vi "Consumer.vi"(8 "error in (no error)":errorcluster, 9 "Data":variant, 10 "Case ID":string, 11 "Monkey in":refnum<class "Monkey.lvclass">) -> (0 "error out":errorcluster, 3 "Monkey out":refnum<class "Monkey.lvclass">)   [LabVIEW 2020, in "TALOS.lvlib" / "Monkey.lvlib" / "Monkey.lvclass"]
uses:
  Monkey.lvclass
  C:/LabVIEW Code/TALOS/talos/Ancestor/Ancestor/Ancestor.lvclass
  C:/LabVIEW Code/TALOS/talos/Father of all uServices/Father of all uServices/Father of all uServices.lvclass
  Monkey Consumer Case Selector.ctl
  Interfaces/Analysis Framework/Analysis Framework.lvclass
  Ancestor/Ancestor/Ancestor.lvclass/Ancestor.ctl
  Father of all uServices/Father of all uServices/Father of all uServices.lvclass/Father of all uServices.ctl
  Monkey.lvclass/Monkey.ctl
  Run Utilities/TypeDefs/Messages/Schedule Message.ctl
  Run Utilities/TypeDefs/DAQ Control.ctl
  Run Utilities/Schedule/Schedule.lvclass
  Father of all uServices/Father of all uServices Messages/Consumer Msg/Consumer Msg.lvclass/Consumer Msg.ctl
  Run Utilities/TypeDefs/Script Checker Result.ctl
  Run Utilities/TypeDefs/Messages/Script Checker Message.ctl
  Guardian/Guardian Messages/Message to uService Msg/Message to uService Msg.lvclass/Message to uService Msg.ctl
  Run Utilities/TypeDefs/Messages/Submit Message.ctl
  Run Utilities/Run Instance/Run Instance.lvclass
  Run Utilities/TypeDefs/Monkey Status.ctl
  Run Utilities/TypeDefs/Messages/Banana Message.ctl
  Run Utilities/TypeDefs/Return Code.ctl
  Inner stop message.ctl
  Ancestor/Ancestor/Read ID.vi
  Guardian/Guardian Messages/Message to uService Msg/Send Message to uService.vi
  FGV/Error Memory/Get Error Description.vi
  Support VIs/Get PC name.vi
  Support VIs/Get Class Name.vi
  FGV/Error Memory/Error Memory Core.vi
  <vilib>/AdvancedString/Delimited String to 1D String Array.vi
  Support VIs/Circus Root Path.vi
  FGV/Error Memory/Error Crt Lvl checker.vi
  FGV/Error Memory/Error Memory Core.vi/40c8088d-b597-4017-91af-faa98e00292e.vi
  FGV/Error Memory/Error Memory Core.vi/d4a3ab98-063c-4e44-b43d-fbdcfe6c2be2.vi
  Father of all uServices/Father of all uServices/Father of all uServices.lvclass
  C:/LabVIEW Code/TALOS/builds/Actor Framework PPL/Actor Framework.lvlibp/1abvi3w/vi.lib/ActorFramework/Actor/Actor.lvclass
  Run Utilities/Optimiser Cell/Optimiser Cell.lvclass
  C:/LabVIEW Code/TALOS/talos/Run Utilities/Cell/Schedule Cell.lvclass
  Support VIs/Global Memory.vi
  <vilib>/Utility/LVClass/Get LV Class Name.vi
  Support VIs/Is in Packed Library.vi
  Support VIs/TALOS Root path.vi
  Support VIs/Read CSV worksheet.vi
  Support VIs/Global Constants.vi
  <vilib>/Utility/error.llb/General Error Handler.vi
  <vilib>/Utility/config.llb/Open Config Data.vi
  <vilib>/Utility/config.llb/Get Section Names.vi
  <vilib>/Utility/config.llb/Get Key Names.vi
  <vilib>/Utility/config.llb/Read Key.vi
  <vilib>/Utility/config.llb/Read Key (String).vi
  <vilib>/Utility/config.llb/Close Config Data.vi
  <vilib>/Utility/error.llb/Search and Replace Pattern.vi
  Support VIs/Error Log.vi
  builds/Actor Framework PPL/Actor Framework.lvlibp/1abvi3w/vi.lib/ActorFramework/Actor/Read Self Enqueuer.vi
  <userlib>/_OpenG.lib/lvdata/lvdata.llb/Get Strings from Enum__ogtk.vi
  builds/Actor Framework PPL/Actor Framework.lvlibp/1abvi3w/vi.lib/ActorFramework/Message Enqueuer/Enqueue.vi
  builds/Actor Framework PPL/Actor Framework.lvlibp/1abvi3w/vi.lib/ActorFramework/Actor/Read Caller Enqueuer.vi
  Father of all uServices/Father of all uServices/Children Methods/Get GUI Item Value - String.vi
  Father of all uServices/Father of all uServices/Multiline string updater.vi
  Ancestor/Ancestor/Ancestor.lvclass
  <vilib>/Comparison/Equal/Equal Functor/Equal Functor.lvclass
  Father of all uServices/Father of all uServices Messages/Consumer Msg/Consumer Msg.lvclass
  Run Utilities/Run Block/Run Block.lvclass
  Guardian/Guardian Messages/Message to uService Msg/Message to uService Msg.lvclass
  TALOS.lvlib
  Run Utilities/Run Utilities.lvlib
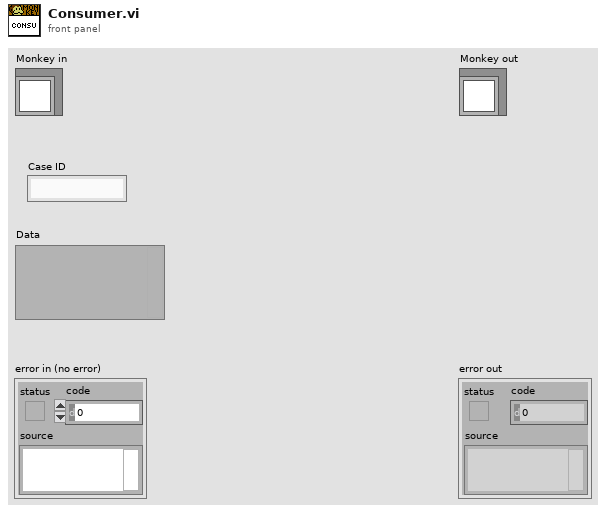
[diagram p1: front panel]
types:
  T1 = typedef "TALOS.lvlib/Monkey.lvlib/Monkey.lvclass/Monkey Consumer Case Selector.ctl" = enum16{"Init", "Update GUI", "New schedule", "Check Script", "Submit Script", "Banana arrived", "Optimiser - evaluate RUN", "Optimiser - update RUN", "Quality Check", "What to do next", "Update Crit Lvl", "Skip Run", "Stop Schedule", "Skip schedule"}
  T2 = cluster{"Font Name:":string, "Size":i16, "Strikeout?":bool, "Italic?":bool, "Underline?":bool, "Outline?":bool, "Shadow?":bool, "Bold?":bool}
  T3 = enum16{"User-specified Font", "Application Font", "System Font", "Dialog Font"}
  T4 = typedef "TALOS.lvlib/Run Utilities.lvlib/Schedule Message.ctl" = cluster{"uS Name":string, "Synchronised":bool, "DAQ Control":T5, "Schedule":refnum<class "Schedule.lvclass">}
  T5 = typedef "TALOS.lvlib/Run Utilities.lvlib/DAQ Control.ctl" = enum16{"On", "Off", "External"}
  T6 = typedef "TALOS.lvlib/Run Utilities.lvlib/Script Checker Message.ctl" = cluster{"Monkey ID":string, "Script Checker Result":T7}
  T7 = typedef "TALOS.lvlib/Run Utilities.lvlib/Script Checker Result.ctl" = enum16{"Passed", "Failed", "Empty"}
  T8 = typedef "TALOS.lvlib/Run Utilities.lvlib/Monkey Status.ctl" = enum16{"Init", "Paused", "Ongoing", "Stopped", "Finished (no errors)", "Finished (with errors)"}
  T9 = typedef "TALOS.lvlib/Run Utilities.lvlib/Submit Message.ctl" = cluster{"DAQ Control":T5, "Run Instance":refnum<class "Run Instance.lvclass">}
  T10 = typedef "TALOS.lvlib/Run Utilities.lvlib/Banana Message.ctl" = cluster{"FPGA Name":string, "Return Code":T11}
  T11 = typedef "TALOS.lvlib/Run Utilities.lvlib/Return Code.ctl" = enum16{"All Good", "Retry", "Skip", "Skip All", "ABORT"}
  T12 = cluster{"left":i16, "top":i16, "right":i16, "bottom":i16}
  T13 = typedef "TALOS.lvlib/Run Utilities.lvlib/Run Instance.lvclass/Run Instance - GUI.ctl" = cluster{"Script Name":string, "Parameters":string[][], "FPGA Name":string}
  T14 = typedef "TALOS.lvlib/Run Utilities.lvlib/Schedule.lvclass/Array of Runs - GUI.ctl" = T15[]
  T15 = typedef "TALOS.lvlib/Run Utilities.lvlib/Schedule Cell.lvclass/Cell - GUI.ctl" = cluster{"Background Color":u32, "Number of cycles":u32, "Single RUN":T13, "Quality check":bool, "Cell Type":string}
  T16 = typedef "TALOS.lvlib/Monkey.lvlib/Monkey.lvclass/Inner stop message.ctl" = cluster{"Old value":bool, "Gracefully?":bool}
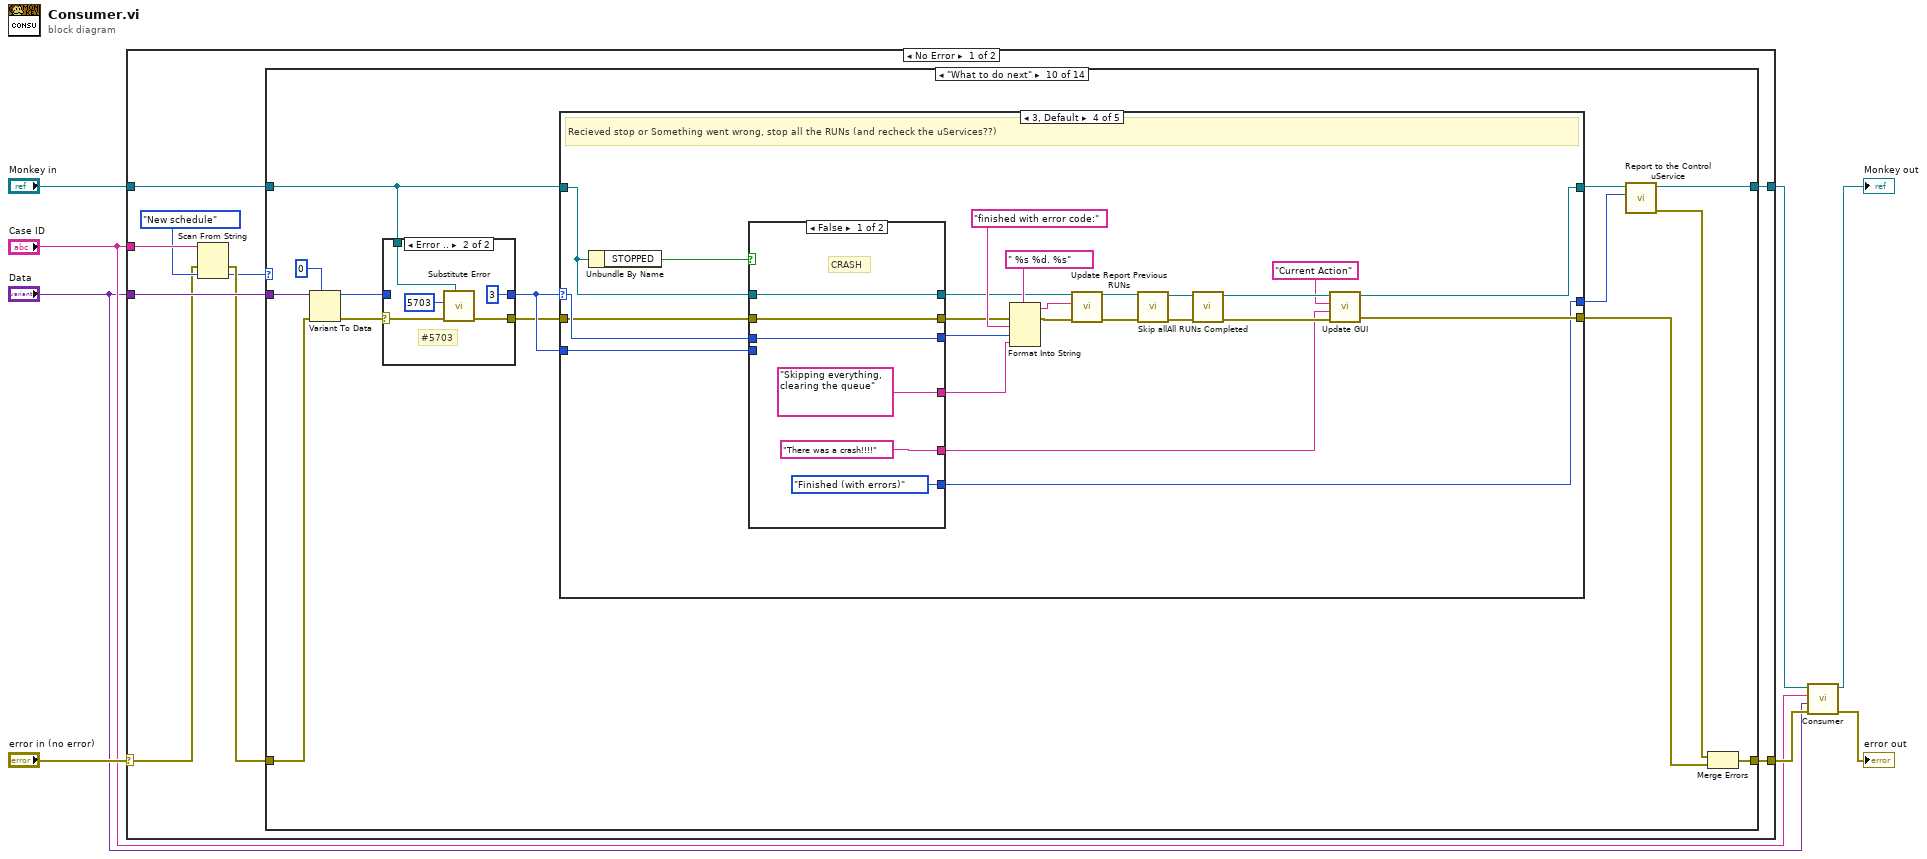
[diagram p0: block diagram]
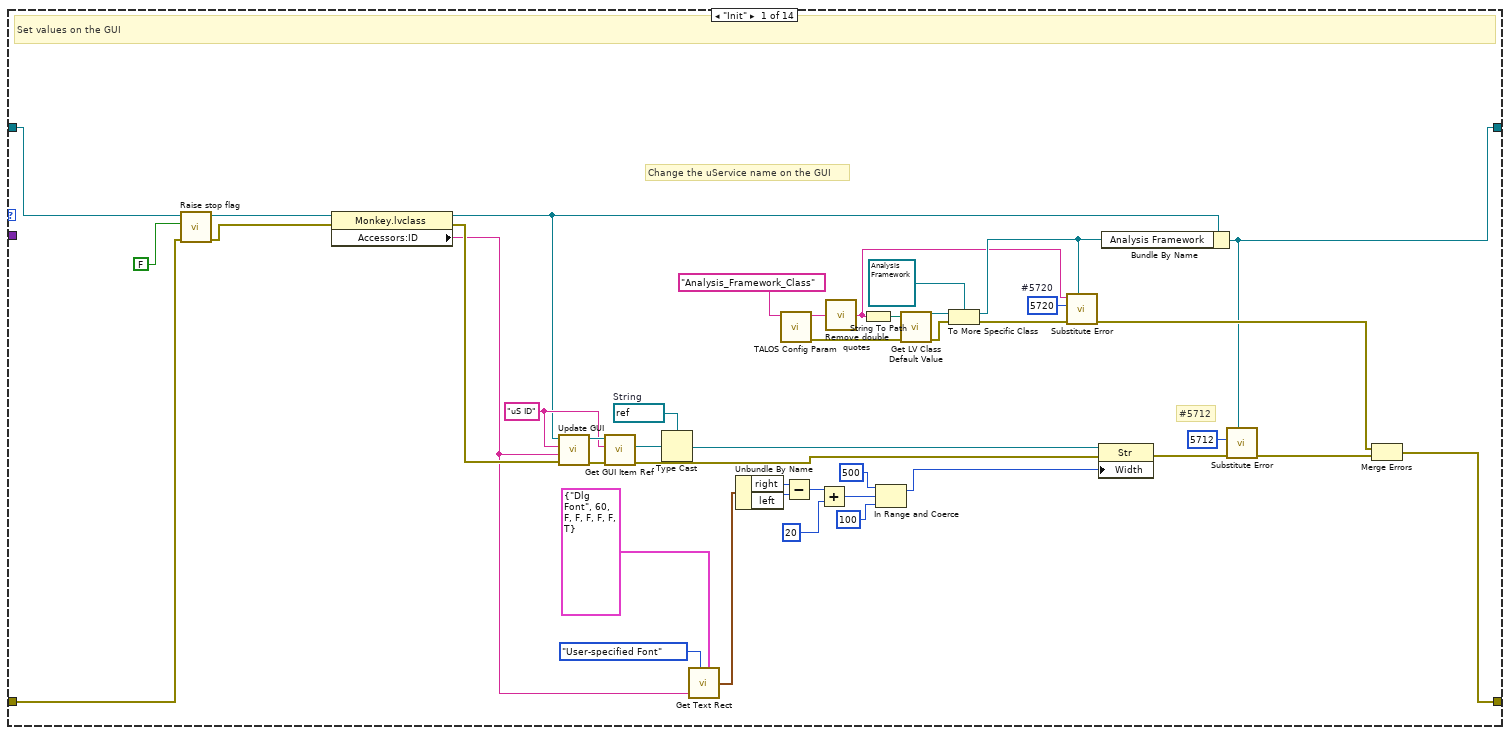
[diagram p2: hidden frame]
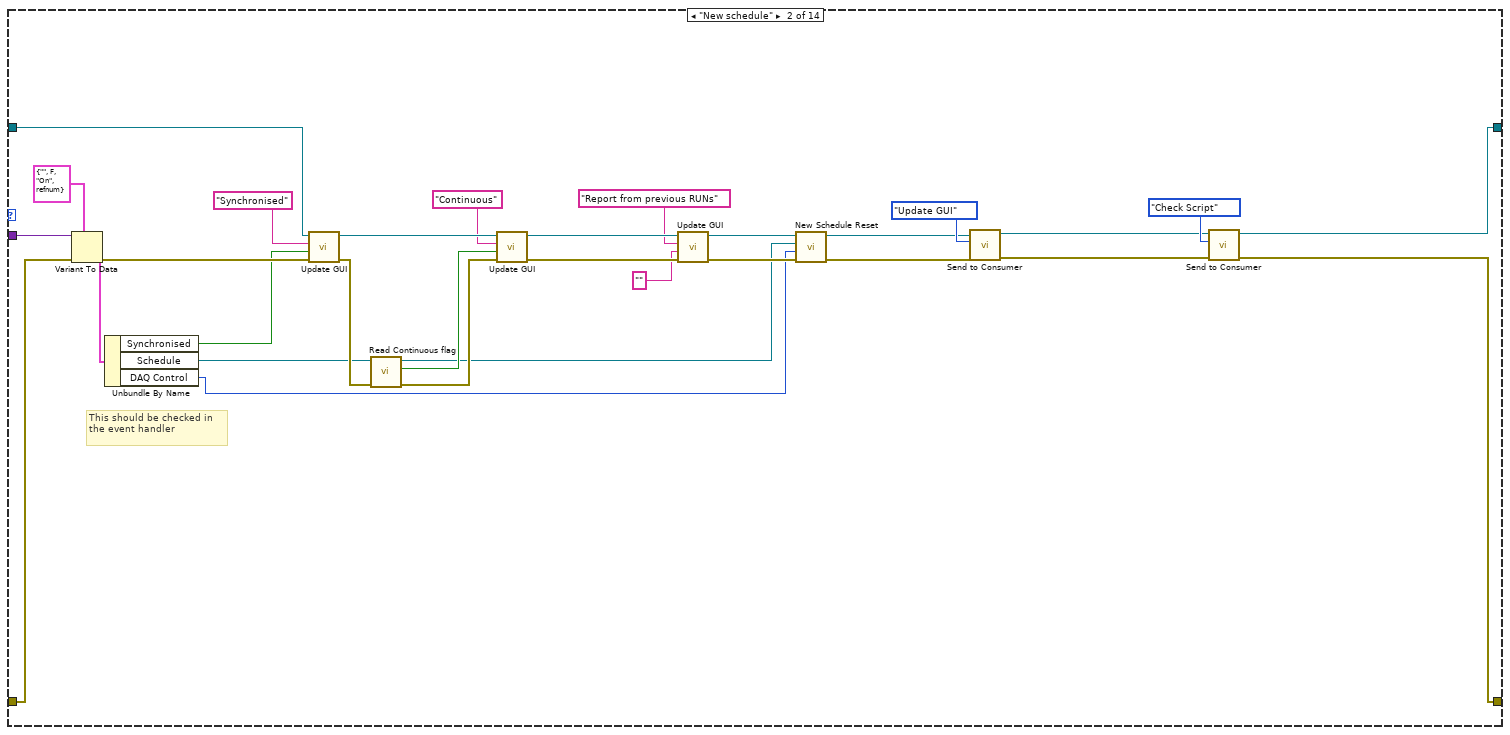
[diagram p3: hidden frame]
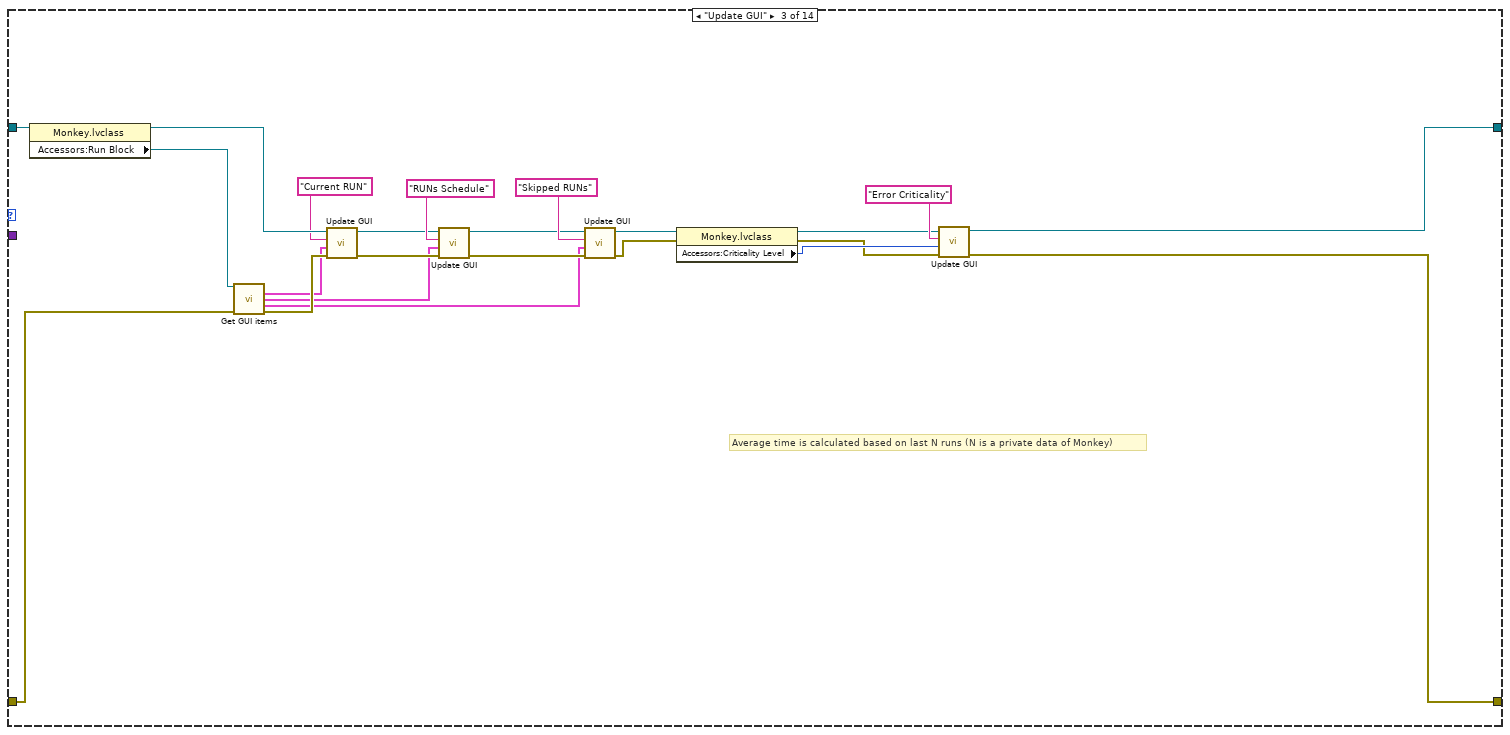
[diagram p4: hidden frame]
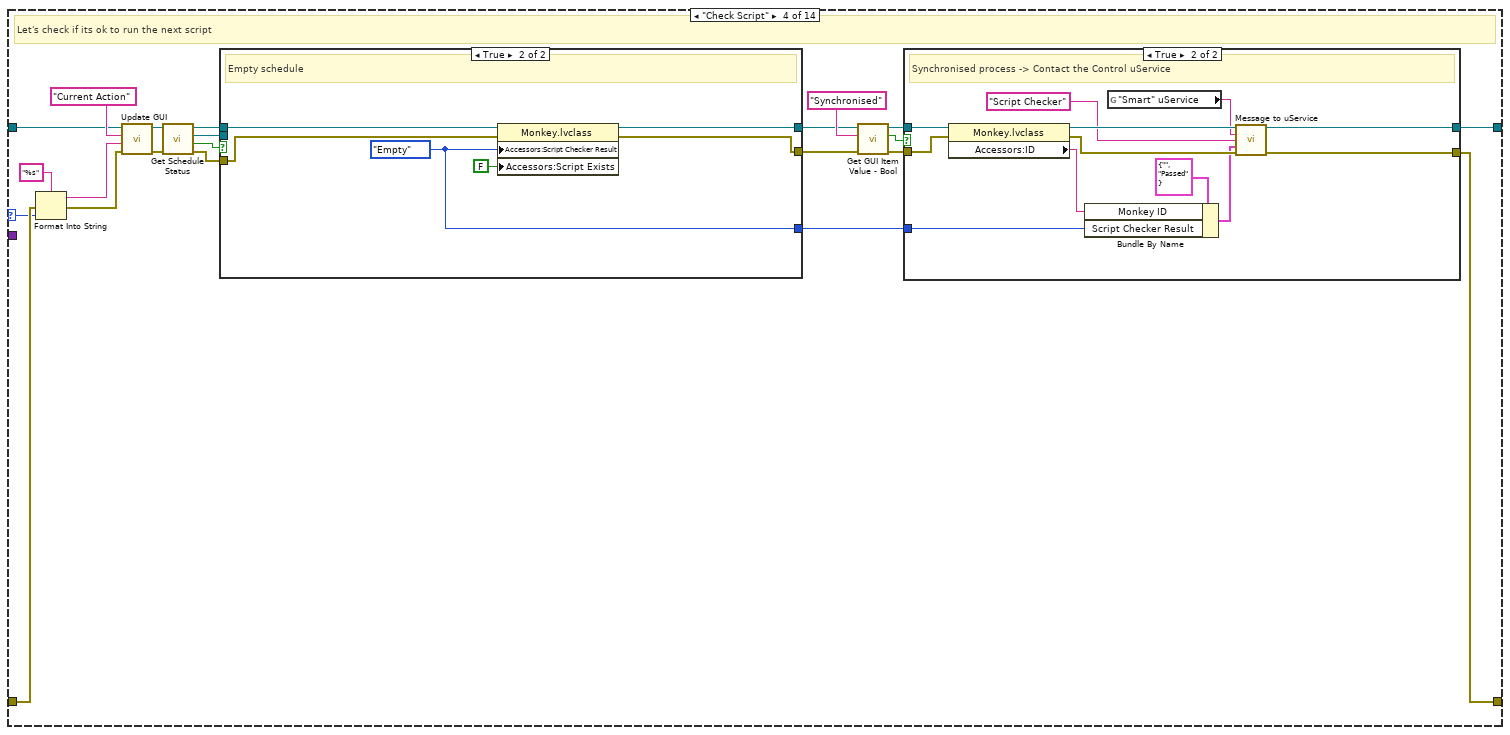
[diagram p5: hidden frame]
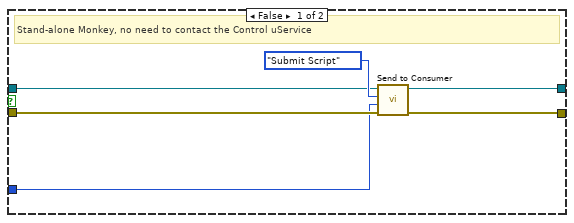
[diagram p6: hidden frame]
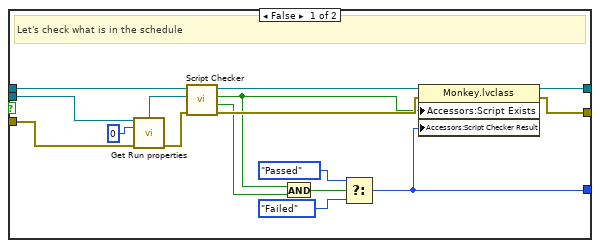
[diagram p7: hidden frame]
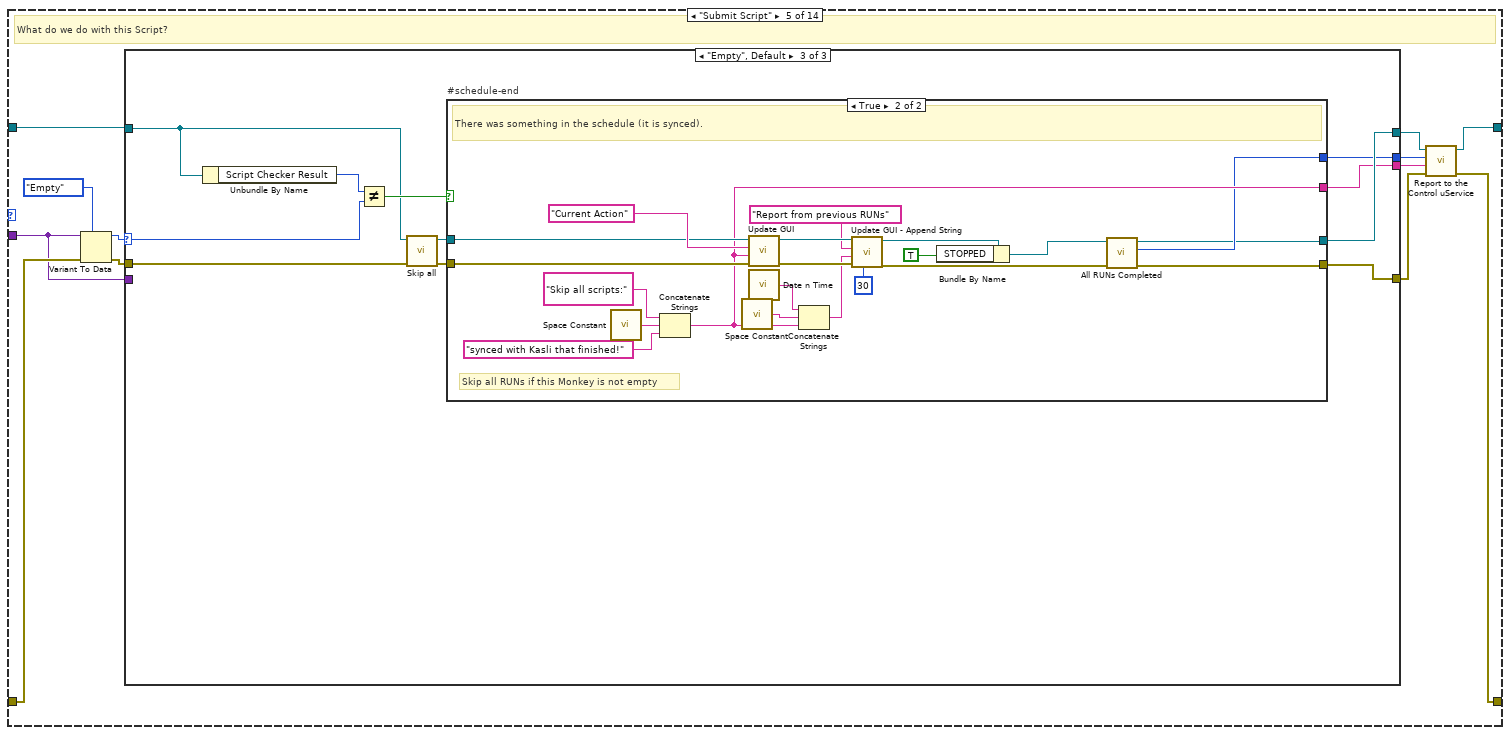
[diagram p8: hidden frame]
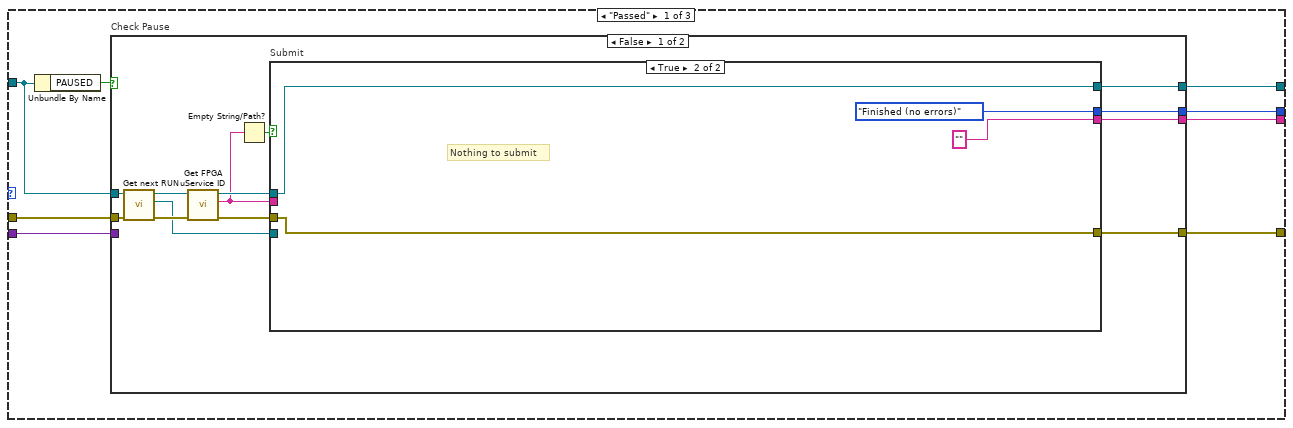
[diagram p9: hidden frame]
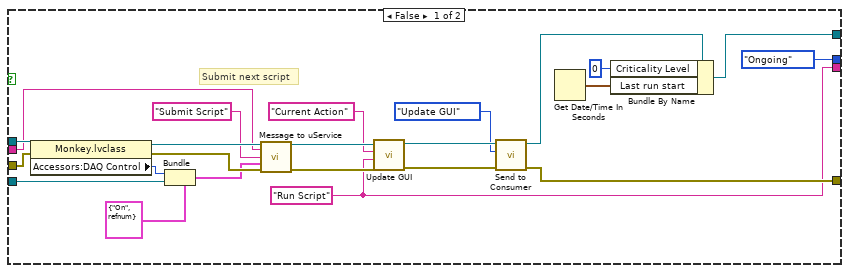
[diagram p10: hidden frame]
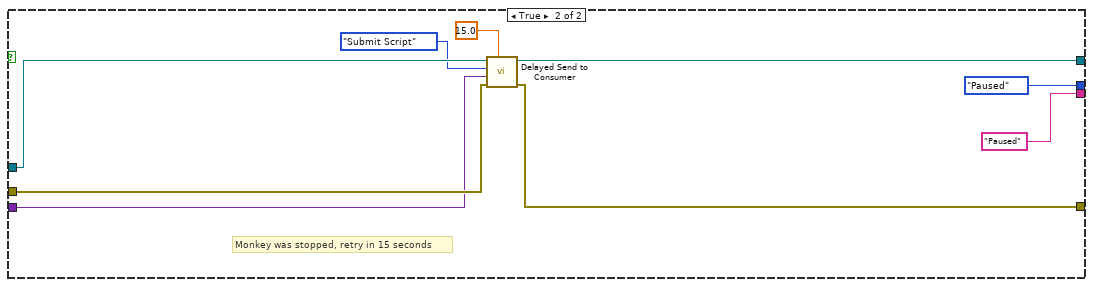
[diagram p11: hidden frame]
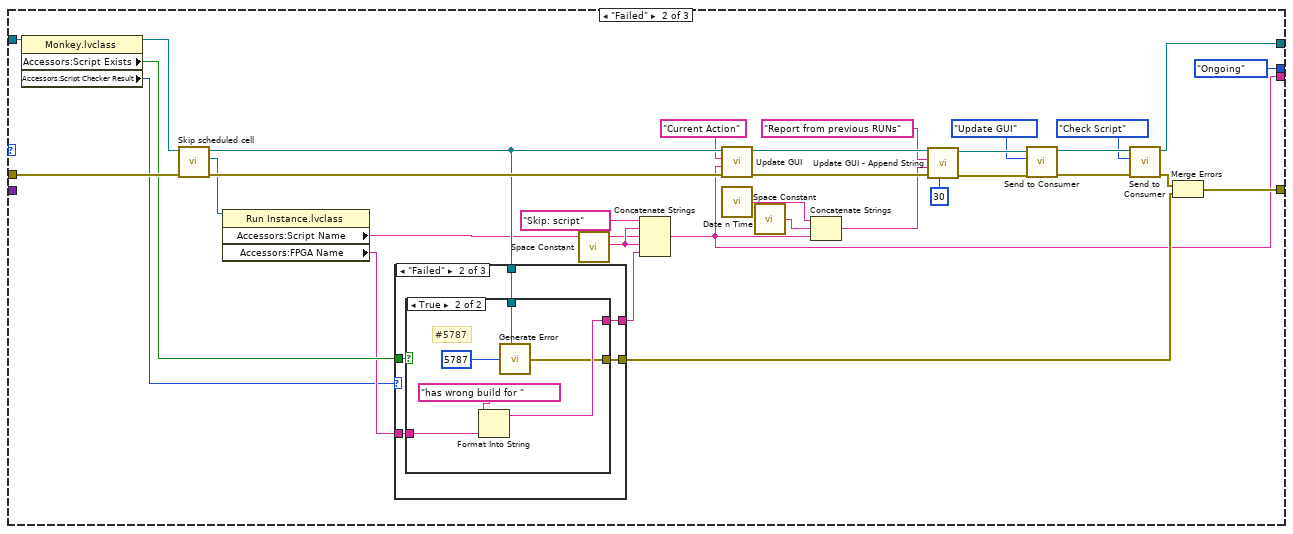
[diagram p12: hidden frame]
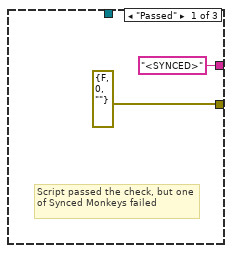
[diagram p13: hidden frame]
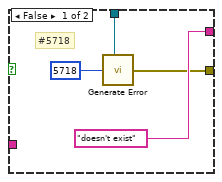
[diagram p14: hidden frame]
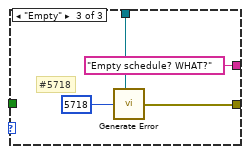
[diagram p15: hidden frame]
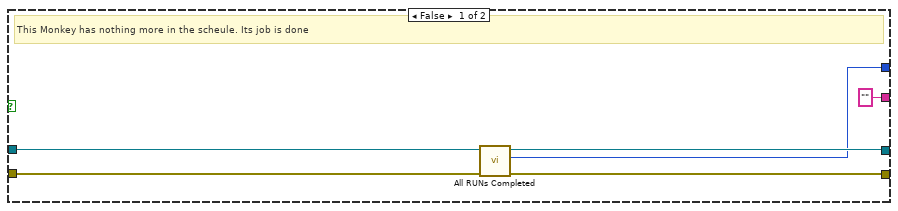
[diagram p16: hidden frame]
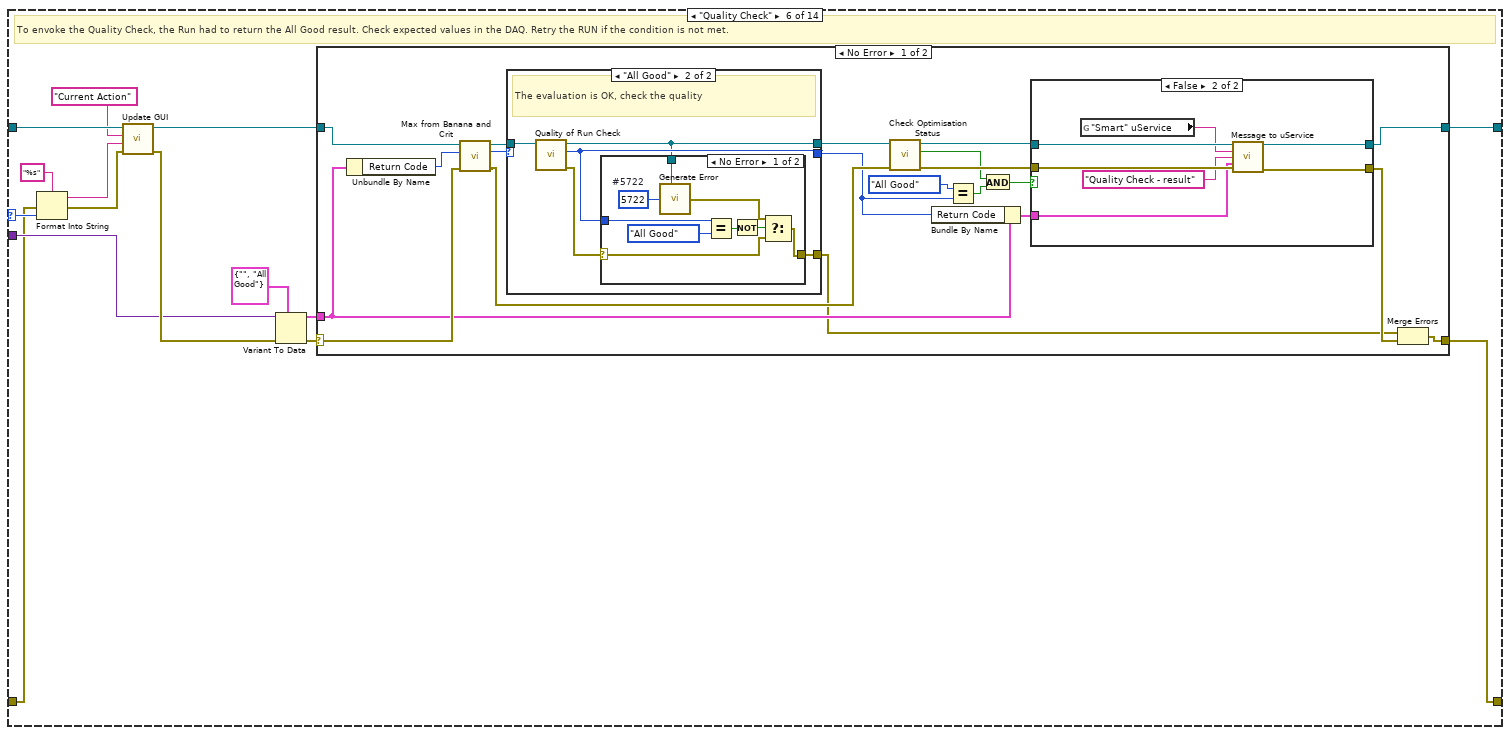
[diagram p17: hidden frame]
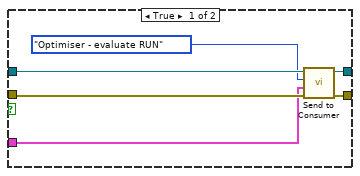
[diagram p18: hidden frame]
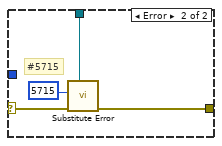
[diagram p20: hidden frame]
diagram:
  n1 = case shown="No Error" "error in (no error)" {
    selector: "error in (no error)" -> [w11 w975]
    tunnel: [w16 w976] -> w3
    tunnel: "Monkey in" -> [w17 w976]
    tunnel: [w14 w975] -> w6
    tunnel: "Case ID" -> [w13 _]
    tunnel: "Data" -> [w15 _]
    frame No Error {
      n2 = Scan From String(input string=w13, error in=w11, default 1=Monkey_Consumer_Case_Selector."New schedule" ("Consumer Case Selector")) -> (error out=w10:errorcluster, output 1=w9:T1)  [unwired: 2 in, 2 out]
      n3 = case shown="\"What to do next\"" w9 {
        selector: w9 -> [_ _ _ w114 _ w342 _ _ _ _ _ _ _ _]
        tunnel: w17 -> [w25 w78 w108 w116 w187 w350 w431 w523 w598 w627 w845 w880 w920 w974]
        tunnel: [w27 w62 w98 w125 w181 w348 w429 w520 w600 w629 w855 w883 w929 w964] -> w16
        tunnel: w15 -> [_ w87 _ _ w176 w349 w428 w519 w596 w631 w860 w884 w930 _]
        tunnel: [w30 w61 w97 w124 w179 w337 w430 w521 w599 w628 w854 w882 w928 w965] -> w14
        tunnel: w10 -> [w23 w84 w111 w118 w186 w339 w432 w522 w597 w630 w859 w890 w932 w973]
        frame "Init" {
          w32 = 5720  # #5720
          w55 = refnum<vi> refnum  # String
          w58 = "uS ID" ("GUI Item Name")
          # "Change the uService name on the GUI"
          # "#5712"
          # "Set values on the GUI"
          n4 = call-dynamic "Raise stop flag.vi"("error in (no error)"=w23, "on/off"=FALSE ("value"), "Monkey in"=w25) -> ("error out"=w24:errorcluster, "Monkey out"=w26:refnum<class "Monkey.lvclass">)  [unwired: 7 in]
          n5 = property class="Monkey.lvclass"(reference=w26, error in=w24) -> (reference out=w28:refnum<class "Monkey.lvclass">, error out=w53:errorcluster, "Accessors:ID"=w47:string)
          n6 = call "Update GUI.vi"("error in (no error)"=w53, "Data"=w47, "GUI Item Name"=w58, "uService Template in"=w28) -> ("error out"=w57:errorcluster, "uService Template out"=w59:refnum<class "Monkey.lvclass">)  [unwired: 6 in]
          n7 = call "Get GUI Item Ref.vi"("error in (no error)"=w57, "FP Item Name"=w58, "uService Template in"=w59) -> ("error out"=w51:errorcluster, "Ctl Refnum"=w56:refnum<vi>)  [unwired: 6 in, 1 out]
          n8 = Type Cast(type=w55, x=w56) -> (*(type *) &x=w52:refnum<vi>)
          n9 = call <vilib>:"Get Text Rect.vi"("desired font(Application)"=T3."User-specified Font", "text"=w47, "[user-specified font]"=T2 {"Font Name:"="Dlg Font", "Size"=60, "Strikeout?"=FALSE, "Italic?"=FALSE, "Underline?"=FALSE, "Outline?"=FALSE, "Shadow?"=FALSE, "Bold?"=TRUE}) -> ("rect"=w48:T12)  [unwired: 6 in]
          n10 = Unbundle By Name(w48) -> ("right"=w46:i16, "left"=w45:i16)
          n11 = call "TALOS Config Param.vi"("Parameter Name"="Analysis_Framework_Class") -> ("error out"=w20:errorcluster, "Output"=w19:string)  [unwired: 9 in]
          n12 = Subtract(x=w46, y=w45) -> (x-y=w44:i16)
          n13 = Add(x=w44, y=i16 20) -> (x+y=w41:i16)
          n14 = call "Remove double quotes.vi"("Input string"=w19) -> ("Output string"=w21:string)  [unwired: 4 in]
          n15 = String To Path(string=w21) -> (path=w37:path)
          n16 = In Range and Coerce(upper limit=i16 500, x=w41, lower limit=i16 100) -> (coerced(x)=w38:i16)  [unwired: 1 out]
          n17 = call <vilib>:"Get LV Class Default Value.vi"("error in (no error)"=w20, "class path"=w37) -> ("error out"=w36:errorcluster, "object"=w35:refnum<class>)  [unwired: 8 in]
          n18 = To More Specific Class(target class=refnum<class "Analysis Framework.lvclass"> refnum ("Analysis Framework"), reference=w35, error in=w36) -> (specific class reference=w29:refnum<class "Analysis Framework.lvclass">, error out=w33:errorcluster)
          n19 = call "Substitute Error.vi"("LabVIEW Object"=w29, "error in (no error)"=w33, "Error Code"=w32, "Optional String"=w21) -> ("error out"=w60:errorcluster)  [unwired: 7 in]
          n20 = property class="Str"(reference=w52, error in=w51, "Width"=w38) -> (error out=w42:errorcluster)  [unwired: 1 out]
          n21 = Bundle By Name(cluster=w28, "Analysis Framework"=w29) -> (w27:refnum<class "Monkey.lvclass">)
          n22 = call "Substitute Error.vi"("LabVIEW Object"=w27, "error in (no error)"=w42, "Error Code"=5712) -> ("error out"=w31:errorcluster)  [unwired: 8 in]
          n23 = Merge Errors(w60, w31) -> (w30:errorcluster)
        }
        frame "New schedule" {
          # "This should be checked in the event handler"
          n24 = Variant To Data(error in=w84, type=T4 {"uS Name"="", "Synchronised"=FALSE, "DAQ Control"=enum."On", "Schedule"=refnum} ("Monkey Schedule Message"), Variant=w87) -> (data=w85:T4, error out=w90:errorcluster)
          n25 = Unbundle By Name(w85) -> ("Synchronised"=w79:bool, "Schedule"=w72:refnum<class "Schedule.lvclass">, "DAQ Control"=w64:T5)
          n26 = call "Update GUI.vi"("error in (no error)"=w90, "Data"=w79, "GUI Item Name"="Synchronised", "uService Template in"=w78) -> ("error out"=w73:errorcluster, "uService Template out"=w82:refnum<class "Monkey.lvclass">)  [unwired: 6 in]
          n27 = call-dynamic "Read Continuous flag.vi"("error in (no error)"=w73, "Schedule in"=w72) -> ("error out"=w88:errorcluster, "Continuous flag"=w81:bool, "Schedule out"=w65:refnum<class "Schedule.lvclass">)  [unwired: 7 in]
          n28 = call "Update GUI.vi"("error in (no error)"=w88, "Data"=w81, "GUI Item Name"="Continuous", "uService Template in"=w82) -> ("error out"=w77:errorcluster, "uService Template out"=w76:refnum<class "Monkey.lvclass">)  [unwired: 6 in]
          n29 = call "Update GUI.vi"("error in (no error)"=w77, "Data"="", "GUI Item Name"="Report from previous RUNs", "uService Template in"=w76) -> ("error out"=w89:errorcluster, "uService Template out"=w67:refnum<class "Monkey.lvclass">)  [unwired: 6 in]
          n30 = call-dynamic "New Schedule Reset.vi"("error in (no error)"=w89, "DAQ Control"=w64, "Schedule"=w65, "Monkey in"=w67) -> ("error out"=w63:errorcluster, "Monkey out"=w66:refnum<class "Monkey.lvclass">)  [unwired: 6 in]
          n31 = call "Send to Consumer.vi"("error in (no error)"=w63, "Case ID"=Monkey_Consumer_Case_Selector."Update GUI" ("Monkey Consumer Case Selector"), "uService Template in"=w66) -> ("error out"=w68:errorcluster, "uService Template out"=w69:refnum<class "Monkey.lvclass">)  [unwired: 7 in]
          n32 = call "Send to Consumer.vi"("error in (no error)"=w68, "Case ID"=Monkey_Consumer_Case_Selector."Check Script" ("Monkey Consumer Case Selector"), "uService Template in"=w69) -> ("error out"=w61:errorcluster, "uService Template out"=w62:refnum<class "Monkey.lvclass">)  [unwired: 7 in]
        }
        frame "Update GUI" {
          # "Average time is calculated based on last N runs (N is a private data of Monkey)"
          n33 = property class="Monkey.lvclass"(reference=w108) -> (reference out=w102:refnum<class "Monkey.lvclass">, "Accessors:Run Block"=w99:refnum<class "Run Block.lvclass">)  [unwired: 1 in, 1 out]
          n34 = call-dynamic "Get GUI items.vi"("Run Block in"=w99, "error in (no error)"=w111) -> ("Current RUN"=w100:T13, "Schedule"=w107:T14, "Skipped RUNs"=w104:T14, "error out"=w110:errorcluster)  [unwired: 9 in, 1 out]
          n35 = call "Update GUI.vi"("error in (no error)"=w110, "Data"=w100, "GUI Item Name"="Current RUN", "uService Template in"=w102) -> ("error out"=w112:errorcluster, "uService Template out"=w103:refnum<class "Monkey.lvclass">)  [unwired: 6 in]
          n36 = call "Update GUI.vi"("error in (no error)"=w112, "Data"=w107, "GUI Item Name"="RUNs Schedule", "uService Template in"=w103) -> ("error out"=w113:errorcluster, "uService Template out"=w105:refnum<class "Monkey.lvclass">)  [unwired: 6 in]
          n37 = call "Update GUI.vi"("error in (no error)"=w113, "Data"=w104, "GUI Item Name"="Skipped RUNs", "uService Template in"=w105) -> ("error out"=w93:errorcluster, "uService Template out"=w94:refnum<class "Monkey.lvclass">)  [unwired: 6 in]
          n38 = property class="Monkey.lvclass"(reference=w94, error in=w93) -> (reference out=w92:refnum<class "Monkey.lvclass">, error out=w91:errorcluster, "Accessors:Criticality Level"=w95:u8)
          n39 = call "Update GUI.vi"("error in (no error)"=w91, "Data"=w95, "GUI Item Name"="Error Criticality", "uService Template in"=w92) -> ("error out"=w97:errorcluster, "uService Template out"=w98:refnum<class "Monkey.lvclass">)  [unwired: 6 in]
        }
        frame "Check Script" {
          # "Let's check if its ok to run the next script"
          n40 = Format Into String(format string="%s", error in=w118, w114) -> (resulting string=w121:string, error out=w119:errorcluster)  [unwired: 1 in]
          n41 = call "Update GUI.vi"("error in (no error)"=w119, "Data"=w121, "GUI Item Name"="Current Action", "uService Template in"=w116) -> ("error out"=w117:errorcluster, "uService Template out"=w115:refnum<class "Monkey.lvclass">)  [unwired: 6 in]
          n42 = call-dynamic "Get Schedule Status.vi"("error in (no error)"=w117, "Monkey in"=w115) -> ("error out"=w135:errorcluster, "Empty?"=w134:bool, "Schedule out"=w133:refnum<class "Schedule.lvclass">, "Monkey out"=w123:refnum<class "Monkey.lvclass">)  [unwired: 6 in]
          n43 = case shown="True" w134 {
            tunnel: w123 -> [w164 w175]
            tunnel: w135 -> [w167 w172]
            tunnel: w133 -> [w166 _]
            tunnel: [w158 w174] -> w131
            tunnel: [w157 w171] -> w128
            tunnel: [w155 w170] -> w126
            frame False {
              # "Let's check what is in the schedule"
              n44 = call "Get Run properties.vi"("Schedule in"=w166, "index"=0, "error in (no error)"=w167) -> ("Run Instance"=w154:refnum<class "Run Instance.lvclass">, "error out"=w168:errorcluster)  [unwired: 5 in, 6 out]
              n45 = call "Script Checker.vi"("error in (no error)"=w168, "Run"=w154, "Monkey in"=w164) -> ("error out"=w169:errorcluster, "Correct Build?"=w162:bool, "Script exists?"=w156:bool, "Monkey out"=w163:refnum<class "Monkey.lvclass">)  [unwired: 5 in]
              n46 = And(x=w156, y=w162) -> (x .and. y?=w159:bool)
              n47 = Select(t=Script_Checker_Result."Passed" ("Script Checker Result"), s=w159, f=Script_Checker_Result."Failed" ("Script Checker Result")) -> (s? t:f=w155:T7)
              n48 = property class="Monkey.lvclass"(reference=w163, error in=w169, "Accessors:Script Exists"=w156, "Accessors:Script Checker Result"=w155) -> (reference out=w158:refnum<class "Monkey.lvclass">, error out=w157:errorcluster)
            }
            frame True {
              w170 = Script_Checker_Result."Empty" ("Script Checker Result")
              # "Empty schedule"
              n49 = property class="Monkey.lvclass"(reference=w175, error in=w172, "Accessors:Script Checker Result"=w170, "Accessors:Script Exists"=FALSE ("Script Exists")) -> (reference out=w174:refnum<class "Monkey.lvclass">, error out=w171:errorcluster)
            }
          }
          n50 = call "Get GUI Item Value - Bool.vi"("error in (no error)"=w128, "FP Item Name"="Synchronised", "uService Template in"=w131) -> ("error out"=w127:errorcluster, "Value"=w129:bool, "uService Template out"=w130:refnum<class "Monkey.lvclass">)  [unwired: 6 in]
          n51 = case shown="True" w129 {
            tunnel: w130 -> [w139 w153]
            tunnel: w127 -> [w141 w150]
            tunnel: w126 -> [w136 w145]
            tunnel: [w138 w144] -> w125
            tunnel: [w137 w143] -> w124
            frame False {
              # "Stand-alone Monkey, no need to contact the Control uService"
              n52 = call "Send to Consumer.vi"("error in (no error)"=w141, "Data"=w136, "Case ID"=Monkey_Consumer_Case_Selector."Submit Script" ("Monkey Consumer Case Selector"), "uService Template in"=w139) -> ("error out"=w137:errorcluster, "uService Template out"=w138:refnum<class "Monkey.lvclass">)  [unwired: 6 in]
            }
            frame True {
              # "Synchronised process -> Contact the Control uService"
              n53 = property class="Monkey.lvclass"(reference=w153, error in=w150) -> (reference out=w152:refnum<class "Monkey.lvclass">, error out=w151:errorcluster, "Accessors:ID"=w148:string)
              n54 = Bundle By Name(cluster=T6 {"Monkey ID"="", "Script Checker Result"=enum."Passed"} ("Message"), "Monkey ID"=w148, "Script Checker Result"=w145) -> (w147:T6)
              n55 = global read "Global Constants.vi" "\"Smart\" uService"() -> (w142:string)
              n56 = call "Message to uService.vi"("Father of all uServices in"=w152, "uService ID"=w142, "Message"="Script Checker", "Data"=w147, "error in (no error)"=w151) -> ("Father of all uServices out"=w144:refnum<class "Monkey.lvclass">, "error out"=w143:errorcluster)  [unwired: 9 in]
            }
          }
        }
        frame "Submit Script" {
          # "What do we do with this Script?"
          n57 = Variant To Data(error in=w186, type=Script_Checker_Result."Empty" ("Script Checker Result"), Variant=w176) -> (data=w183:T7, error out=w185:errorcluster)
          n58 = case shown="\"Empty\", Default" w183 {
            selector: w183 -> [_ _ w308]
            tunnel: w187 -> [w190 w257 w304]
            tunnel: w185 -> [w191 w256 w303]
            tunnel: [w194 w255 w302] -> w182
            tunnel: [w195 w254 w301] -> w180
            tunnel: [w193 Monkey_Status."Ongoing" ("Monkey Status") w300] -> w178
            tunnel: [w192 w245 w299] -> w177
            tunnel: w176 -> [w188 _ _]
            frame "Passed" {
              n59 = Unbundle By Name(w190) -> ("PAUSED"=w189:bool)
              n60 = case "Check Pause" shown="False" w189 {
                tunnel: [w206 w239] -> w195
                tunnel: [w205 w241] -> w194
                tunnel: [w204 Monkey_Status."Paused" ("Monkey Status")] -> w193
                tunnel: [w203 "Paused"] -> w192
                tunnel: w191 -> [w199 w240]
                tunnel: w190 -> [w196 w242]
                tunnel: w188 -> [_ w237]
                frame False {
                  n61 = call "Get next RUN.vi"("error in (no error)"=w199, "Monkey in"=w196) -> ("error out"=w208:errorcluster, "Current RUN"=w207:refnum<class "Run Instance.lvclass">, "Monkey out"=w202:refnum<class "Monkey.lvclass">)  [unwired: 7 in]
                  n62 = call-dynamic "Get FPGA uService ID.vi"("error in (no error)"=w208, "Monkey in"=w202) -> ("error out"=w200:errorcluster, "FPGA uService ID"=w197:string, "Monkey out"=w201:refnum<class "Monkey.lvclass">)  [unwired: 7 in]
                  n63 = Empty String/Path?(string/path=w197) -> (empty?=w198:bool)
                  n64 = case "Submit" shown="True" w198 {
                    tunnel: w207 -> [w228 _]
                    tunnel: [w220 w234] -> w206
                    tunnel: [w215 w235] -> w205
                    tunnel: [Monkey_Status."Ongoing" ("Monkey Status") Monkey_Status."Finished (no errors)" ("Monkey Status")] -> w204
                    tunnel: [w213 ""] -> w203
                    tunnel: w201 -> [w211 w235]
                    tunnel: w200 -> [w210 w234]
                    tunnel: w197 -> [w209 _]
                    frame False {
                      w213 = "Run Script"
                      # "Submit next script"
                      n65 = property class="Monkey.lvclass"(reference=w211, error in=w210) -> (reference out=w227:refnum<class "Monkey.lvclass">, error out=w230:errorcluster, "Accessors:DAQ Control"=w226:T5)
                      n66 = Bundle(cluster=T9 {"DAQ Control"=enum."On", "Run Instance"=refnum} ("Submit Msg"), "DAQ Control"=w226, "Run Instance"=w228) -> (w225:T9)
                      n67 = call "Message to uService.vi"("Father of all uServices in"=w227, "uService ID"=w209, "Message"="Submit Script", "Data"=w225, "error in (no error)"=w230) -> ("Father of all uServices out"=w224:refnum<class "Monkey.lvclass">, "error out"=w223:errorcluster)  [unwired: 9 in]
                      n68 = call "Update GUI.vi"("error in (no error)"=w223, "Data"=w213, "GUI Item Name"="Current Action", "uService Template in"=w224) -> ("error out"=w221:errorcluster, "uService Template out"=w231:refnum<class "Monkey.lvclass">)  [unwired: 6 in]
                      n69 = call "Send to Consumer.vi"("error in (no error)"=w221, "Case ID"=Monkey_Consumer_Case_Selector."Update GUI" ("Monkey Consumer Case Selector"), "uService Template in"=w231) -> ("error out"=w220:errorcluster, "uService Template out"=w218:refnum<class "Monkey.lvclass">)  [unwired: 7 in]
                      n70 = Get Date/Time In Seconds() -> (seconds since 1Jan1904=w216:timestamp)
                      n71 = Bundle By Name(cluster=w218, "Criticality Level"=u8 0, "Last run start"=w216) -> (w215:refnum<class "Monkey.lvclass">)
                    }
                    frame True {
                      # "Nothing to submit"
                    }
                  }
                }
                frame True {
                  # "Monkey was stopped, retry in 15 seconds"
                  n72 = call "Delayed Send to Consumer.vi"("Seconds (5)"=15.0, "error in (no error)"=w240, "Data"=w237, "Case ID"=Monkey_Consumer_Case_Selector."Submit Script" ("Monkey Consumer Case Selector"), "Father of all uServices in"=w242) -> ("error out"=w239:errorcluster, "Father of all uServices out"=w241:refnum<class "Monkey.lvclass">)  [unwired: 5 in]
                }
              }
            }
            frame "Failed" {
              n73 = property class="Monkey.lvclass"(reference=w257) -> (reference out=w252:refnum<class "Monkey.lvclass">, "Accessors:Script Exists"=w253:bool, "Accessors:Script Checker Result"=w247:T7)  [unwired: 1 in, 1 out]
              n74 = call-dynamic "Skip scheduled cell.vi"("error in (no error)"=w256, "Monkey in"=w252) -> ("error out"=w277:errorcluster, "Skipped Run"=w251:refnum<class "Run Instance.lvclass">, "Monkey out"=w276:refnum<class "Monkey.lvclass">)  [unwired: 7 in]
              n75 = property class="Run Instance.lvclass"(reference=w251) -> ("Accessors:Script Name"=w250:string, "Accessors:FPGA Name"=w249:string)  [unwired: 1 in, 2 out]
              n76 = case shown="\"Failed\"" w247 {
                tunnel: ["<SYNCED>" w284 "Empty schedule? WHAT?"] -> w260
                tunnel: [errorcluster {"status"=FALSE, "code"=0, "source"=""} ("error out") w283 w296] -> w259
                tunnel: w253 -> [_ w282 _]
                tunnel: w249 -> [_ w281 _]
                tunnel: w276 -> [_ w280 w295]
                frame "Passed" {
                  # "Script passed the check, but one of Synced Monkeys failed"
                }
                frame "Failed" {
                  n77 = case shown="True" w282 {
                    tunnel: w281 -> [_ w294]
                    tunnel: w280 -> [w287 w291]
                    tunnel: ["doesn't exist" w290] -> w284
                    tunnel: [w285 w289] -> w283
                    frame False {
                      # "#5718"
                      n78 = call "Generate Error.vi"("Class"=w287, "Error Code"=5718) -> ("error out"=w285:errorcluster)  [unwired: 5 in]
                    }
                    frame True {
                      # "#5787"
                      n79 = Format Into String(initial string="has wrong build for " ("t"), w294) -> (resulting string=w290:string)  [unwired: 2 in, 1 out]
                      n80 = call "Generate Error.vi"("Class"=w291, "Error Code"=5787) -> ("error out"=w289:errorcluster)  [unwired: 5 in]
                    }
                  }
                }
                frame "Empty" {
                  # "#5718"
                  n81 = call "Generate Error.vi"("Class"=w295, "Error Code"=5718) -> ("error out"=w296:errorcluster)  [unwired: 5 in]
                }
              }
              n82 = call <vilib>:"Space Constant.vi"() -> ("String"=w266:string)
              n83 = Concatenate Strings("Skip: script" ("GUI Item Name"), w266, w250, w266, w260) -> (w245:string)
              n84 = call "Update GUI.vi"("error in (no error)"=w277, "Data"=w245, "GUI Item Name"="Current Action", "uService Template in"=w276) -> ("error out"=w271:errorcluster, "uService Template out"=w272:refnum<class "Monkey.lvclass">)  [unwired: 6 in]
              n85 = call "Date n Time.vi"() -> ("Date & Time"=w262:string)  [unwired: 5 in]
              n86 = call <vilib>:"Space Constant.vi"() -> ("String"=w263:string)
              n87 = Concatenate Strings(w262, w263, w245) -> (w261:string)
              n88 = call "Update GUI - Append String.vi"("Lines to keep"=u8 30, "error in (no error)"=w271, "String"=w261, "GUI Item Name"="Report from previous RUNs", "Father of all uServices in"=w272) -> ("error out"=w273:errorcluster, "Father of all uServices out"=w275:refnum<class "Monkey.lvclass">)  [unwired: 5 in]
              n89 = call "Send to Consumer.vi"("error in (no error)"=w273, "Case ID"=Monkey_Consumer_Case_Selector."Update GUI" ("Monkey Consumer Case Selector"), "uService Template in"=w275) -> ("error out"=w268:errorcluster, "uService Template out"=w274:refnum<class "Monkey.lvclass">)  [unwired: 7 in]
              n90 = call "Send to Consumer.vi"("error in (no error)"=w268, "Case ID"=Monkey_Consumer_Case_Selector."Check Script" ("Monkey Consumer Case Selector"), "uService Template in"=w274) -> ("error out"=w258:errorcluster, "uService Template out"=w255:refnum<class "Monkey.lvclass">)  [unwired: 7 in]
              n91 = Merge Errors(w258, w259) -> (w254:errorcluster)
            }
            frame "Empty", Default {
              n92 = Unbundle By Name(w304) -> ("Script Checker Result"=w309:T7)
              n93 = Not Equal?(x=w309, y=w308) -> (x != y?=w307:bool)
              n94 = call-dynamic "Skip all.vi"("error in (no error)"=w303, "Monkey in"=w304) -> ("error out"=w306:errorcluster, "Monkey out"=w305:refnum<class "Monkey.lvclass">)  [unwired: 8 in]
              n95 = case "#schedule-end" shown="True" w307 {
                tunnel: w306 -> [w311 w325]
                tunnel: [w313 w316] -> w302
                tunnel: [w312 w317] -> w301
                tunnel: w305 -> [w314 w324]
                tunnel: [w310 w318] -> w300
                tunnel: ["" w321] -> w299
                frame False {
                  # "This Monkey has nothing more in the scheule. Its job is done"
                  n96 = call-dynamic "All RUNs Completed.vi"("error in (no error)"=w311, "Monkey in"=w314) -> ("error out"=w312:errorcluster, "Monkey Status"=w310:T8, "Monkey out"=w313:refnum<class "Monkey.lvclass">)  [unwired: 7 in]
                }
                frame True {
                  # "Skip all RUNs if this Monkey is not empty"
                  # "There was something in the schedule (it is synced)."
                  n97 = call <vilib>:"Space Constant.vi"() -> ("String"=w332:string)
                  n98 = Concatenate Strings("Skip all scripts:" ("GUI Item Name"), w332, "synced with Kasli that finished!" ("string")) -> (w321:string)
                  n99 = call <vilib>:"Space Constant.vi"() -> ("String"=w329:string)
                  n100 = call "Update GUI.vi"("error in (no error)"=w325, "Data"=w321, "GUI Item Name"="Current Action", "uService Template in"=w324) -> ("error out"=w335:errorcluster, "uService Template out"=w336:refnum<class "Monkey.lvclass">)  [unwired: 6 in]
                  n101 = call "Date n Time.vi"() -> ("Date & Time"=w328:string)  [unwired: 5 in]
                  n102 = Concatenate Strings(w328, w329, w321) -> (w327:string)
                  n103 = call "Update GUI - Append String.vi"("Lines to keep"=u8 30, "error in (no error)"=w335, "String"=w327, "GUI Item Name"="Report from previous RUNs", "Father of all uServices in"=w336) -> ("error out"=w319:errorcluster, "Father of all uServices out"=w323:refnum<class "Monkey.lvclass">)  [unwired: 5 in]
                  n104 = Bundle By Name(cluster=w323, "STOPPED"=TRUE) -> (w320:refnum<class "Monkey.lvclass">)
                  n105 = call-dynamic "All RUNs Completed.vi"("error in (no error)"=w319, "Monkey in"=w320) -> ("error out"=w317:errorcluster, "Monkey Status"=w318:T8, "Monkey out"=w316:refnum<class "Monkey.lvclass">)  [unwired: 7 in]
                }
              }
            }
          }
          n106 = call-dynamic "Report to the Control uService.vi"("error in (no error)"=w180, "Current Action"=w177, "Monkey Status"=w178, "Monkey in"=w182) -> ("error out"=w179:errorcluster, "Monkey out"=w181:refnum<class "Monkey.lvclass">)  [unwired: 6 in]
        }
        frame "Quality Check" {
          # "To envoke the Quality Check, the Run had to return the All Good result. Check expected values in the DAQ. Retry the RUN if the condition is not met."
          n107 = Format Into String(format string="%s", error in=w339, w342) -> (resulting string=w341:string, error out=w338:errorcluster)  [unwired: 1 in]
          n108 = call "Update GUI.vi"("error in (no error)"=w338, "Data"=w341, "GUI Item Name"="Current Action", "uService Template in"=w350) -> ("error out"=w351:errorcluster, "uService Template out"=w343:refnum<class "Monkey.lvclass">)  [unwired: 6 in]
          n109 = Variant To Data(error in=w351, type=T10 {"FPGA Name"="", "Return Code"=enum."All Good"} ("Cluster"), Variant=w349) -> (data=w346:T10, error out=w345:errorcluster)
          n110 = case shown="No Error" w345 {
            selector: w345 -> [w369 w416]
            tunnel: [w354 w413] -> w348
            tunnel: [w353 w408] -> w337
            tunnel: w343 -> [w371 w409]
            tunnel: w346 -> [w366 _]
            frame No Error {
              n111 = Unbundle By Name(w366) -> ("Return Code"=w368:T11)
              n112 = call-dynamic "Max from Banana and Crit.vi"("error in (no error)"=w369, "Return Code"=w368, "Monkey in"=w371) -> ("error out"=w356:errorcluster, "Return Code"=w367:T11, "Monkey out"=w370:refnum<class "Monkey.lvclass">)  [unwired: 6 in]
              n113 = case shown="\"All Good\"" w367 {
                selector: w367 -> [w385 _]
                tunnel: w370 -> [w386 w391]
                tunnel: [w386 w388] -> w363
                tunnel: [w385 w390] -> w355
                tunnel: [_ w387] -> w352
                frame Default {
                  # "The overall result is higher than 0"
                }
                frame "All Good" {
                  # "The evaluation is OK, check the quality"
                  n114 = call-dynamic "Quality of Run Check.vi"("Monkey in"=w391) -> ("error out"=w389:errorcluster, "Check Result"=w390:T11, "Monkey out"=w388:refnum<class "Monkey.lvclass">)  [unwired: 8 in]
                  n115 = case shown="No Error" w389 {
                    selector: w389 -> [w394 w402]
                    tunnel: w390 -> [w400 _]
                    tunnel: w388 -> [w398 w403]
                    tunnel: [w393 w401] -> w387
                    frame No Error {
                      w392 = 5722  # #5722
                      n116 = call "Generate Error.vi"("Class"=w398, "Error Code"=w392) -> ("error out"=w395:errorcluster)  [unwired: 5 in]
                      n117 = Equal?(x=w400, y=Return_Code."All Good" ("x")) -> (x = y?=w397:bool)
                      n118 = Not(x=w397) -> (.not. x?=w396:bool)
                      n119 = Select(t=w395, s=w396, f=w394) -> (s? t:f=w393:errorcluster)
                    }
                    frame Error {
                      # "#5715"
                      n120 = call "Substitute Error.vi"("LabVIEW Object"=w403, "error in (no error)"=w402, "Error Code"=5715) -> ("error out"=w401:errorcluster)  [unwired: 8 in]
                    }
                  }
                }
              }
              n121 = call-dynamic "Check Optimisation Status.vi"("error in (no error)"=w356, "Monkey in"=w363) -> ("error out"=w361:errorcluster, "Optimiser"=w358:bool, "Monkey out"=w362:refnum<class "Monkey.lvclass">)  [unwired: 7 in]
              n122 = Bundle By Name(cluster=w366, "Return Code"=w355) -> (w365:T10)
              n123 = Equal?(x=Return_Code."All Good", y=w355) -> (x = y?=w359:bool)
              n124 = And(x=w358, y=w359) -> (x .and. y?=w357:bool)
              n125 = case shown="False" w357 {
                tunnel: w362 -> [w375 w384]
                tunnel: w361 -> [w377 w383]
                tunnel: [w376 w379] -> w354
                tunnel: [w372 w378] -> w364
                tunnel: w365 -> [w373 w380]
                frame True {
                  n126 = call "Send to Consumer.vi"("error in (no error)"=w377, "Data"=w373, "Case ID"=Monkey_Consumer_Case_Selector."Optimiser - evaluate RUN" ("Consumer Case Selector"), "uService Template in"=w375) -> ("error out"=w372:errorcluster, "uService Template out"=w376:refnum<class "Monkey.lvclass">)  [unwired: 6 in]
                }
                frame False {
                  n127 = global read "Global Constants.vi" "\"Smart\" uService"() -> (w381:string)
                  n128 = call "Message to uService.vi"("Father of all uServices in"=w384, "uService ID"=w381, "Message"="Quality Check - result", "Data"=w380, "error in (no error)"=w383) -> ("Father of all uServices out"=w379:refnum<class "Monkey.lvclass">, "error out"=w378:errorcluster)  [unwired: 9 in]
                }
              }
              n129 = Merge Errors(w352, w364) -> (w353:errorcluster)
            }
            frame Error {
              # "#5207"
              n130 = call "Substitute Error.vi"("LabVIEW Object"=w409, "error in (no error)"=w416, "Error Code"=5207, "Optional String"="Wrong format of the Banana in Quality Check!") -> ("error out"=w405:errorcluster)  [unwired: 7 in]
              n131 = global read "Global Constants.vi" "\"Smart\" uService"() -> (w407:string)
              n132 = property class="Monkey.lvclass"(reference=w409) -> (reference out=w412:refnum<class "Monkey.lvclass">, "Accessors:ID"=w411:string)  [unwired: 1 in, 1 out]
              n133 = call "Message to uService.vi"("Father of all uServices in"=w412, "uService ID"=w407, "Message"=" Quality Check - result", "Data"=w411) -> ("Father of all uServices out"=w413:refnum<class "Monkey.lvclass">, "error out"=w406:errorcluster)  [unwired: 10 in]
              n134 = Merge Errors(w405, w406) -> (w408:errorcluster)
            }
          }
        }
        frame "Optimiser - evaluate RUN" {
          n135 = call "Update GUI.vi"("error in (no error)"=w432, "Data"="Optimiser" ("GUI Item Name"), "GUI Item Name"="Current Action", "uService Template in"=w431) -> ("error out"=w418:errorcluster, "uService Template out"=w419:refnum<class "Monkey.lvclass">)  [unwired: 6 in]
          n136 = property class="Monkey.lvclass"(reference=w419, error in=w418) -> (reference out=w423:refnum<class "Monkey.lvclass">, error out=w424:errorcluster, "Accessors:Run Block"=w420:refnum<class "Run Block.lvclass">, "Accessors:Analysis Framework"=w417:refnum<class "Analysis Framework.lvclass">)
          n137 = call-dynamic "Get Optimiser Cell.vi"("error in (no error)"=w424, "Run Block in"=w420) -> ("error out"=w427:errorcluster, "Optimiser Cell"=w421:refnum<class "Optimiser Cell.lvclass">, "Run Block out"=w422:refnum<class "Run Block.lvclass">)  [unwired: 7 in]
          n138 = case shown="No Error" w427 {
            selector: w427 -> [w445 w506]
            tunnel: w423 -> [w453 w510]
            tunnel: w422 -> [w452 _]
            tunnel: w421 -> [w451 _]
            tunnel: w417 -> [w446 _]
            tunnel: [w438 w509] -> w429
            tunnel: w428 -> [w435 w508]
            tunnel: [w443 w507] -> w430
            frame No Error {
              # "#5713"
              n139 = call-dynamic "Calculate Observables.vi"("Analysis Framework"=w446, "error in (no error)"=w445, "Optimiser Cell in"=w451) -> ("error out"=w450:errorcluster, "Retry?"=w448:bool, "Optimiser Cell out"=w449:refnum<class "Optimiser Cell.lvclass">)  [unwired: 6 in]
              n140 = case shown="No Error" w450 {
                selector: w450 -> [w480 w504]
                tunnel: w449 -> [w482 w503]
                tunnel: w448 -> [w483 _]
                tunnel: [w481 w503] -> w447
                tunnel: [w478 _] -> w437
                tunnel: [w477 w502] -> w436
                tunnel: [w479 w504] -> w441
                tunnel: w435 -> [w476 w502]
                tunnel: [w475 _] -> w433
                frame No Error {
                  n141 = case shown="True" w483 {
                    tunnel: w482 -> [w488 w500]
                    tunnel: [w485 w500] -> w481
                    tunnel: w480 -> [w487 w493]
                    tunnel: [w486 w501] -> w479
                    tunnel: [Monkey_Consumer_Case_Selector."Optimiser - update RUN" ("Monkey Consumer Case Selector") Monkey_Consumer_Case_Selector."Optimiser - evaluate RUN" ("Monkey Consumer Case Selector")] -> w478
                    tunnel: [w484 w499] -> w477
                    tunnel: w476 -> [w484 w499]
                    tunnel: [_ w497] -> w475
                    frame False {
                      # "Observables calculated properly, ask optimiser for new set of parameters"
                      n142 = call-dynamic "Reset NaN Retries Counter.vi"("error in (no error)"=w487, "Run Optimiser in"=w488) -> ("error out"=w486:errorcluster, "Run Optimiser out"=w485:refnum<class "Optimiser Cell.lvclass">)  [unwired: 8 in]
                    }
                    frame True {
                      w494 = 5716  # #5716
                      # "NaN encountered, try reading the observable again"
                      n143 = call "TALOS Config Param.vi"("error in (no error)"=w493, "Parameter Name"="Optimiser_Wait_s") -> ("error out"=w492:errorcluster, "Output"=w490:string)  [unwired: 8 in]
                      n144 = Scan From String(input string=w490, error in=w492, default 1=5.0 ("default value 1")) -> (error out=w496:errorcluster, output 1=w497:dbl)  [unwired: 2 in, 2 out]
                      n145 = call "Substitute Error.vi"("LabVIEW Object"=w500, "error in (no error)"=w496, "Error Code"=w494) -> ("error out"=w501:errorcluster)  [unwired: 8 in]
                    }
                  }
                }
                frame Error {
                }
              }
              n146 = call-dynamic "Replace Scheduled Cell.vi"("Schedule Cell"=w447, "Run Block in"=w452) -> ("error out"=w442:errorcluster, "Run Block out"=w454:refnum<class "Run Block.lvclass">)  [unwired: 8 in]
              n147 = property class="Monkey.lvclass"(reference=w453, "Accessors:Run Block"=w454) -> (reference out=w439:refnum<class "Monkey.lvclass">)  [unwired: 1 in, 1 out]
              n148 = Merge Errors(w442, w441) -> (w440:errorcluster)
              n149 = case shown="No Error" w440 {
                selector: w440 -> [w459 w464]
                tunnel: w439 -> [w461 w474]
                tunnel: [w460 w471] -> w438
                tunnel: w437 -> [w458 _]
                tunnel: w436 -> [w457 w466]
                tunnel: [w456 w463] -> w434
                tunnel: w433 -> [w455 _]
                frame No Error {
                  n150 = call "Delayed Send to Consumer.vi"("Seconds (5)"=w455, "error in (no error)"=w459, "Data"=w457, "Case ID"=w458, "Father of all uServices in"=w461) -> ("error out"=w456:errorcluster, "Father of all uServices out"=w460:refnum<class "Monkey.lvclass">)  [unwired: 5 in]
                }
                frame Error {
                  # "If there was an error we want to skip this because something is wrong with the optimiser"
                  n151 = Variant To Data(type=T10 {"FPGA Name"="", "Return Code"=enum."All Good"} ("Cluster"), Variant=w466) -> (data=w469:T10, error out=w462:errorcluster)  [unwired: 1 in]
                  n152 = global read "Global Constants.vi" "\"Smart\" uService"() -> (w473:string)
                  n153 = Bundle By Name(cluster=w469, "Return Code"=Return_Code."Skip") -> (w468:T10)
                  n154 = call "Message to uService.vi"("Father of all uServices in"=w474, "uService ID"=w473, "Message"="Quality Check - result", "Data"=w468) -> ("Father of all uServices out"=w471:refnum<class "Monkey.lvclass">, "error out"=w465:errorcluster)  [unwired: 10 in]
                  n155 = Merge Errors(w465, w464, w462) -> (w463:errorcluster)
                }
              }
              n156 = call "Substitute Error.vi"("LabVIEW Object"=w438, "error in (no error)"=w434, "Error Code"=5713) -> ("error out"=w443:errorcluster)  [unwired: 8 in]
            }
            frame Error {
              # "Not the optimiser cell, so we can ignore it"
              n157 = call <vilib>:"Clear Errors.vi"("error in (no error)"=w506) -> ("error out"=w505:errorcluster)  [unwired: 5 in, 1 out]
              n158 = global read "Global Constants.vi" "\"Smart\" uService"() -> (w511:string)
              n159 = call "Message to uService.vi"("Father of all uServices in"=w510, "uService ID"=w511, "Message"="Quality Check - result", "Data"=w508, "error in (no error)"=w505) -> ("Father of all uServices out"=w509:refnum<class "Monkey.lvclass">, "error out"=w507:errorcluster)  [unwired: 9 in]
            }
          }
        }
        frame "Optimiser - update RUN" {
          # "Optimiser finished?\nIf it is finished -> remove the schedule cell from the schedule, go to the script checker.\nIf it isn't finished -> Get the new parameters, update the Schedule Cell (with new parameters in the Run Instance), go to the script checker"
          n160 = property class="Monkey.lvclass"(reference=w523) -> (reference out=w518:refnum<class "Monkey.lvclass">, "Accessors:Analysis Framework"=w513:refnum<class "Analysis Framework.lvclass">, "Accessors:Run Block"=w514:refnum<class "Run Block.lvclass">)  [unwired: 1 in, 1 out]
          n161 = call-dynamic "Get Optimiser Cell.vi"("error in (no error)"=w522, "Run Block in"=w514) -> ("error out"=w515:errorcluster, "Optimiser Cell"=w516:refnum<class "Optimiser Cell.lvclass">, "Run Block out"=w517:refnum<class "Run Block.lvclass">)  [unwired: 7 in]
          n162 = case shown="No Error" w515 {
            selector: w515 -> [w540 w594]
            tunnel: w518 -> [w547 w591]
            tunnel: w517 -> [w546 _]
            tunnel: [w525 w589] -> w521
            tunnel: w516 -> [w541 _]
            tunnel: w513 -> [w536 _]
            tunnel: [w532 w590] -> w520
            tunnel: w519 -> [w528 w585]
            frame No Error {
              # "#5714"
              n163 = call-dynamic "Run Optimiser.vi"("Analysis Framework"=w536, "error in (no error)"=w540, "Optimiser Cell in"=w541) -> ("error out"=w537:errorcluster, "Optimiser Cell out"=w538:refnum<class "Optimiser Cell.lvclass">, "Optimiser Finished"=w539:bool)  [unwired: 6 in]
              n164 = call-dynamic "Replace Scheduled Cell.vi"("error in (no error)"=w537, "Schedule Cell"=w538, "Run Block in"=w546) -> ("error out"=w542:errorcluster, "Run Block out"=w545:refnum<class "Run Block.lvclass">)  [unwired: 7 in]
              n165 = property class="Monkey.lvclass"(reference=w547, "Accessors:Run Block"=w545) -> (reference out=w543:refnum<class "Monkey.lvclass">)  [unwired: 1 in, 1 out]
              n166 = case shown="True" w539 {
                tunnel: w543 -> [w552 w571]
                tunnel: [w551 w570] -> w533
                tunnel: w542 -> [w554 w569]
                tunnel: [w553 w578] -> w530
                tunnel: w528 -> [w550 w568]
                tunnel: [w548 w568] -> w524
                tunnel: [errorcluster {"status"=FALSE, "code"=0, "source"=""} ("error out") w566] -> w526
                frame False {
                  # "Optimisation not reached"
                  n167 = case shown="No Error" w554 {
                    selector: w554 -> [w556 w560]
                    tunnel: [w556 w565] -> w553
                    tunnel: w552 -> [w557 w564]
                    tunnel: [w557 w564] -> w551
                    tunnel: w550 -> [w555 w559]
                    tunnel: [w555 w562] -> w548
                    frame No Error {
                    }
                    frame Error {
                      n168 = Variant To Data(error in=w560, type=T10 {"FPGA Name"="", "Return Code"=enum."All Good"} ("Cluster"), Variant=w559) -> (data=w558:T10, error out=w565:errorcluster)
                      n169 = Bundle By Name(cluster=w558, "Return Code"=Return_Code."Skip") -> (w562:T10)
                    }
                  }
                }
                frame True {
                  # "Optimisation reached"
                  n170 = call-dynamic "Run Best Optimisation Parameters.vi"("error in (no error)"=w569, "Monkey in"=w571) -> ("error out"=w578:errorcluster, "Best Parameters"=w567:string[][], "Monkey out"=w570:refnum<class "Monkey.lvclass">)  [unwired: 7 in]
                  n171 = for {
                    tunnel: w567 -> [w581] mode=indexing
                    tunnel: [w579] -> w575 mode=indexing
                    n172 = call <vilib>:"1D String Array to Delimited String.vi"("delimiter"="=", "string array"=w581) -> ("delimited string"=w579:string)  [unwired: 9 in]
                  }
                  n173 = call <vilib>:"1D String Array to Delimited String.vi"("delimiter"="\r", "string array"=w575) -> ("delimited string"=w573:string)  [unwired: 9 in]
                  n174 = Concatenate Strings("Optimiser finished. Best parameters are:\n" ("Text"), w573) -> (w572:string)
                  n175 = call "Temporised Pop-up Window.vi"("Timeout"=5.0, "Text"=w572) -> ("error out"=w566:errorcluster)  [unwired: 9 in]
                }
              }
              n176 = global read "Global Constants.vi" "\"Smart\" uService"() -> (w535:string)
              n177 = call "Message to uService.vi"("Father of all uServices in"=w533, "uService ID"=w535, "Message"="Quality Check - result", "Data"=w524) -> ("Father of all uServices out"=w532:refnum<class "Monkey.lvclass">, "error out"=w531:errorcluster)  [unwired: 10 in]
              n178 = Merge Errors(w531, w530) -> (w529:errorcluster)
              n179 = call "Substitute Error.vi"("LabVIEW Object"=w532, "error in (no error)"=w529, "Error Code"=5714) -> ("error out"=w527:errorcluster)  [unwired: 8 in]
              n180 = Merge Errors(w527, w526) -> (w525:errorcluster)
            }
            frame Error {
              # "Just in case, let the Tamer know that something is up"
              # "Not an optimise cell, this should be impossible to reach"
              n181 = Variant To Data(type=T10 {"FPGA Name"="", "Return Code"=enum."All Good"} ("Cluster"), Variant=w585) -> (data=w586:T10, error out=w582:errorcluster)  [unwired: 1 in]
              n182 = global read "Global Constants.vi" "\"Smart\" uService"() -> (w592:string)
              n183 = Bundle By Name(cluster=w586, "Return Code"=Return_Code."Skip") -> (w584:T10)
              n184 = call "Message to uService.vi"("Father of all uServices in"=w591, "uService ID"=w592, "Message"=" Quality Check - result", "Data"=w584) -> ("Father of all uServices out"=w590:refnum<class "Monkey.lvclass">, "error out"=w583:errorcluster)  [unwired: 10 in]
              n185 = Merge Errors(w583, w582, w594) -> (w589:errorcluster)
            }
          }
        }
        frame "Banana arrived" {
          # "This case is needed to avoid the race condition of an error getting enqueued immediately after the Run is finished: the Monkey would then skip the Criticality Level associated to that error (and, by the way, using it in the subsequent Run). In this way, the \"What to do next\" will be enqued after any - reasonably - possible \"Error Criticality\" message from the Error Manager."
          n186 = call "Send to Consumer.vi"("error in (no error)"=w597, "Data"=w596, "Case ID"=Monkey_Consumer_Case_Selector."What to do next" ("Consumer Case Selector"), "uService Template in"=w598) -> ("error out"=w599:errorcluster, "uService Template out"=w601:refnum<class "Monkey.lvclass">)  [unwired: 6 in]
          n187 = in-place {
            # "Calculate average time per script"
            n188 = in-place-cluster #1(w601) -> ("Last run start"=w607:timestamp, "Times of last N runs"=w610:dbl[], "N"=w605:u32)  [unwired: 1 out]
            n189 = Get Date/Time In Seconds() -> (seconds since 1Jan1904=w611:timestamp)
            n190 = Subtract(x=w611, y=w607) -> (x-y=w609:dbl)
            n191 = Insert Into Array(array=w610, new element=w609) -> (w608:dbl[])  [unwired: 1 in]
            n192 = Array Size(array=w608) -> (size(s)=w613:i32)
            n193 = Greater?(x=w613, y=w605) -> (0:w612:bool)
            n194 = case shown="True" w612 {
              tunnel: w608 -> [w614 w617]
              tunnel: [w614 w615] -> w603
              frame False {
              }
              frame True {
                # "This will be 11th point, remove the first one (oldest)"
                n195 = Delete From Array(array=w617, index=0) -> (array with subset deleted=w615:dbl[])  [unwired: 1 in, 1 out]
              }
            }
            n196 = Array Size(array=w603) -> (size(s)=w602:i32)
            n197 = Add Array Elements(numeric array=w603) -> (sum=w606:dbl)
            n198 = Divide(x=w606, y=w602) -> (x/y=w604:dbl)
            n199 = in-place-cluster #1("Last run start"=w607, "Times of last N runs"=w603, "Average time per script"=w604, "N"=w605) -> (w600:refnum<class "Monkey.lvclass">)
          }
        }
        frame "What to do next" {
          n200 = Variant To Data(error in=w630, type=u16 0, Variant=w631) -> (data=w624:u16, error out=w625:errorcluster)
          n201 = case shown="Error .." w625 {
            selector: w625 -> [w836 w841]
            tunnel: w624 -> [w837 _]
            tunnel: [w837 u16 3] -> w619
            tunnel: [w836 w840] -> w618
            tunnel: w627 -> [_ w838]
            frame No Error {
            }
            frame Error {
              # "#5703"
              n202 = call "Substitute Error.vi"("LabVIEW Object"=w838, "error in (no error)"=w841, "Error Code"=5703) -> ("error out"=w840:errorcluster)  [unwired: 8 in]
            }
          }
          n203 = case shown="3, Default" w619 {
            selector: w619 -> [_ w693 w735 w799 w830]
            tunnel: w618 -> [w639 w695 w737 w793 w823]
            tunnel: w627 -> [w638 w694 w736 w795 w824]
            tunnel: [w643 w690 w729 w791 w825] -> w623
            tunnel: [w644 w689 w728 w790 w822] -> w620
            tunnel: w619 -> [_ _ _ w798 _]
            tunnel: [w640 w683 w731 w787 Monkey_Status."Finished (with errors)" ("Monkey Status")] -> w622
            frame 0 {
              # "All good! Go to the next RUN on the list."
              n204 = call "Update Report Previous RUNs.vi"("error in (no error)"=w639, "Previous RUN outcome"=" finished well!" ("string"), "Monkey in"=w638) -> ("error out"=w635:errorcluster, "Monkey out"=w636:refnum<class "Monkey.lvclass">)  [unwired: 7 in]
              n205 = call-dynamic "The End of the RUN.vi"("error in (no error)"=w635, "Monkey in"=w636) -> ("error out"=w633:errorcluster, "Monkey out"=w634:refnum<class "Monkey.lvclass">)  [unwired: 8 in]
              n206 = call-dynamic "Get Schedule Status.vi"("error in (no error)"=w633, "Monkey in"=w634) -> ("error out"=w637:errorcluster, "Empty?"=w641:bool, "Monkey out"=w642:refnum<class "Monkey.lvclass">)  [unwired: 6 in, 1 out]
              n207 = case shown="False" w641 {
                tunnel: [w653 w667] -> w644
                tunnel: [w652 w668] -> w643
                tunnel: w642 -> [w656 w664]
                tunnel: w637 -> [w647 w665]
                tunnel: [Monkey_Status."Ongoing" ("Monkey Status") w666] -> w640
                frame False {
                  # "More scripts to go"
                  n208 = call "Send to Consumer.vi"("error in (no error)"=w647, "Case ID"=Monkey_Consumer_Case_Selector."Update GUI" ("Consumer Case Selector"), "uService Template in"=w656) -> ("error out"=w645:errorcluster, "uService Template out"=w657:refnum<class "Monkey.lvclass">)  [unwired: 7 in]
                  n209 = call "Send to Consumer.vi"("error in (no error)"=w645, "Case ID"=Monkey_Consumer_Case_Selector."Check Script" ("Consumer Case Selector"), "uService Template in"=w657) -> ("error out"=w655:errorcluster, "uService Template out"=w654:refnum<class "Monkey.lvclass">)  [unwired: 7 in]
                  n210 = call "Update GUI.vi"("error in (no error)"=w655, "Data"="Next RUN!" ("GUI Item Name"), "GUI Item Name"="Current Action", "uService Template in"=w654) -> ("error out"=w653:errorcluster, "uService Template out"=w652:refnum<class "Monkey.lvclass">)  [unwired: 6 in]
                }
                frame True {
                  # "List's empty, means we've finished!"
                  n211 = call "Get GUI Item Value - Bool.vi"("error in (no error)"=w665, "FP Item Name"="Synchronised", "uService Template in"=w664) -> ("error out"=w661:errorcluster, "Value"=w658:bool, "uService Template out"=w662:refnum<class "Monkey.lvclass">)  [unwired: 6 in]
                  n212 = case shown="True" w658 {
                    tunnel: w662 -> [w670 w682]
                    tunnel: w661 -> [w669 w679]
                    tunnel: [w670 w674] -> w660
                    tunnel: [w669 w673] -> w659
                    frame False {
                      # "Stand-alone Monkey, no need to contact the Control uService"
                    }
                    frame True {
                      # "Synchronised process -> Contact the Control uService"
                      n213 = property class="Monkey.lvclass"(reference=w682, error in=w679) -> (reference out=w681:refnum<class "Monkey.lvclass">, error out=w680:errorcluster, "Accessors:ID"=w677:string)
                      n214 = Bundle By Name(cluster=T6 {"Monkey ID"="", "Script Checker Result"=enum."Passed"} ("Message"), "Monkey ID"=w677, "Script Checker Result"=Script_Checker_Result."Empty") -> (w676:T6)
                      n215 = global read "Global Constants.vi" "\"Smart\" uService"() -> (w671:string)
                      n216 = call "Message to uService.vi"("Father of all uServices in"=w681, "uService ID"=w671, "Message"="Script Checker", "Data"=w676, "error in (no error)"=w680) -> ("Father of all uServices out"=w674:refnum<class "Monkey.lvclass">, "error out"=w673:errorcluster)  [unwired: 9 in]
                    }
                  }
                  n217 = call-dynamic "All RUNs Completed.vi"("error in (no error)"=w659, "Monkey in"=w660) -> ("error out"=w667:errorcluster, "Monkey Status"=w666:T8, "Monkey out"=w668:refnum<class "Monkey.lvclass">)  [unwired: 7 in]
                }
              }
            }
            frame 1 {
              # "The RUN didn't go well: re-execute the script"
              n218 = Format Into String(format string=" %s %d. %s", error in=w695, "finished with error code:" ("initial string"), w693, "Retry another time" ("initial string")) -> (resulting string=w699:string, error out=w700:errorcluster)  [unwired: 1 in]
              n219 = call "Update Report Previous RUNs.vi"("error in (no error)"=w700, "Previous RUN outcome"=w699, "Monkey in"=w694) -> ("error out"=w684:errorcluster, "Monkey out"=w685:refnum<class "Monkey.lvclass">)  [unwired: 7 in]
              n220 = Unbundle By Name(w685) -> ("STOPPED"=w687:bool)
              n221 = case shown="False" w687 {
                tunnel: w685 -> [w706 w717]
                tunnel: [w713 w721] -> w691
                tunnel: [w712 w722] -> w688
                tunnel: w684 -> [w705 w716]
                tunnel: ["Next RUN!" ("GUI Item Name") "Runs stopped! Last script finished" ("Text to log")] -> w686
                tunnel: [Monkey_Status."Ongoing" ("Monkey Status") w718] -> w683
                frame False {
                  n222 = call-dynamic "Retry RUN.vi"("error in (no error)"=w705, "Next?"=TRUE, "Monkey in"=w706) -> ("error out"=w704:errorcluster, "Monkey out"=w702:refnum<class "Monkey.lvclass">)  [unwired: 7 in]
                  n223 = call "Send to Consumer.vi"("error in (no error)"=w704, "Case ID"=Monkey_Consumer_Case_Selector."Update GUI" ("Consumer Case Selector"), "uService Template in"=w702) -> ("error out"=w710:errorcluster, "uService Template out"=w701:refnum<class "Monkey.lvclass">)  [unwired: 7 in]
                  n224 = call "Send to Consumer.vi"("error in (no error)"=w710, "Case ID"=Monkey_Consumer_Case_Selector."Check Script" ("Consumer Case Selector"), "uService Template in"=w701) -> ("error out"=w713:errorcluster, "uService Template out"=w712:refnum<class "Monkey.lvclass">)  [unwired: 7 in]
                }
                frame True {
                  n225 = call-dynamic "Skip all.vi"("error in (no error)"=w716, "Monkey in"=w717) -> ("error out"=w714:errorcluster, "Monkey out"=w715:refnum<class "Monkey.lvclass">)  [unwired: 8 in]
                  n226 = call-dynamic "All RUNs Completed.vi"("error in (no error)"=w714, "Monkey in"=w715) -> ("error out"=w719:errorcluster, "Monkey Status"=w718:T8, "Monkey out"=w720:refnum<class "Monkey.lvclass">)  [unwired: 7 in]
                  n227 = call "Send to Consumer.vi"("error in (no error)"=w719, "Case ID"=Monkey_Consumer_Case_Selector."Update GUI" ("Consumer Case Selector"), "uService Template in"=w720) -> ("error out"=w721:errorcluster, "uService Template out"=w722:refnum<class "Monkey.lvclass">)  [unwired: 7 in]
                }
              }
              n228 = call "Update GUI.vi"("error in (no error)"=w691, "Data"=w686, "GUI Item Name"="Current Action", "uService Template in"=w688) -> ("error out"=w689:errorcluster, "uService Template out"=w690:refnum<class "Monkey.lvclass">)  [unwired: 6 in]
            }
            frame 2 {
              # "Skip the Run"
              n229 = Format Into String(format string=" %s %d. %s", error in=w737, "finished with error code:" ("initial string"), w735, "Skipping it and moving to the next one." ("initial string")) -> (resulting string=w741:string, error out=w742:errorcluster)  [unwired: 1 in]
              n230 = call "Update Report Previous RUNs.vi"("error in (no error)"=w742, "Previous RUN outcome"=w741, "Monkey in"=w736) -> ("error out"=w732:errorcluster, "Monkey out"=w733:refnum<class "Monkey.lvclass">)  [unwired: 7 in]
              n231 = Unbundle By Name(w733) -> ("STOPPED"=w734:bool)
              n232 = case shown="True" w734 {
                tunnel: w733 -> [w747 w773]
                tunnel: [w753 w778] -> w727
                tunnel: [w752 w779] -> w730
                tunnel: w732 -> [w744 w772]
                tunnel: [w751 "Runs stopped! Last script finished" ("Text to log")] -> w726
                tunnel: [w743 w775] -> w731
                frame False {
                  n233 = call-dynamic "Skip RUN.vi"("error in (no error)"=w744, "Monkey in"=w747) -> ("error out"=w745:errorcluster, "Monkey out"=w746:refnum<class "Monkey.lvclass">)  [unwired: 8 in]
                  n234 = call-dynamic "Get Schedule Status.vi"("error in (no error)"=w745, "Monkey in"=w746) -> ("error out"=w748:errorcluster, "Empty?"=w750:bool, "Monkey out"=w749:refnum<class "Monkey.lvclass">)  [unwired: 6 in, 1 out]
                  n235 = case shown="False" w750 {
                    tunnel: [w763 w766] -> w753
                    tunnel: [w762 w765] -> w752
                    tunnel: ["Next RUN!" ("GUI Item Name") "All the RUNs completed!" ("Text to log")] -> w751
                    tunnel: w749 -> [w757 w768]
                    tunnel: w748 -> [w760 w767]
                    tunnel: [Monkey_Status."Ongoing" ("Monkey Status") w764] -> w743
                    frame False {
                      # "More scripts to go"
                      n236 = call "Send to Consumer.vi"("error in (no error)"=w760, "Case ID"=Monkey_Consumer_Case_Selector."Update GUI" ("Consumer Case Selector"), "uService Template in"=w757) -> ("error out"=w759:errorcluster, "uService Template out"=w756:refnum<class "Monkey.lvclass">)  [unwired: 7 in]
                      n237 = call "Send to Consumer.vi"("error in (no error)"=w759, "Case ID"=Monkey_Consumer_Case_Selector."Check Script" ("Consumer Case Selector"), "uService Template in"=w756) -> ("error out"=w763:errorcluster, "uService Template out"=w762:refnum<class "Monkey.lvclass">)  [unwired: 7 in]
                    }
                    frame True {
                      # "Empty schedule"
                      n238 = call-dynamic "All RUNs Completed.vi"("error in (no error)"=w767, "Monkey in"=w768) -> ("error out"=w766:errorcluster, "Monkey Status"=w764:T8, "Monkey out"=w765:refnum<class "Monkey.lvclass">)  [unwired: 7 in]
                    }
                  }
                }
                frame True {
                  n239 = call-dynamic "Skip all.vi"("error in (no error)"=w772, "Monkey in"=w773) -> ("error out"=w770:errorcluster, "Monkey out"=w771:refnum<class "Monkey.lvclass">)  [unwired: 8 in]
                  n240 = call-dynamic "All RUNs Completed.vi"("error in (no error)"=w770, "Monkey in"=w771) -> ("error out"=w776:errorcluster, "Monkey Status"=w775:T8, "Monkey out"=w777:refnum<class "Monkey.lvclass">)  [unwired: 7 in]
                  n241 = call "Send to Consumer.vi"("error in (no error)"=w776, "Case ID"=Monkey_Consumer_Case_Selector."Update GUI" ("Consumer Case Selector"), "uService Template in"=w777) -> ("error out"=w778:errorcluster, "uService Template out"=w779:refnum<class "Monkey.lvclass">)  [unwired: 7 in]
                }
              }
              n242 = call "Update GUI.vi"("error in (no error)"=w727, "Data"=w726, "GUI Item Name"="Current Action", "uService Template in"=w730) -> ("error out"=w728:errorcluster, "uService Template out"=w729:refnum<class "Monkey.lvclass">)  [unwired: 6 in]
            }
            frame 3, Default {
              # "Recieved stop or Something went wrong, stop all the RUNs (and recheck the uServices??)"
              n243 = Unbundle By Name(w795) -> ("STOPPED"=w800:bool)
              n244 = case shown="False" w800 {
                tunnel: w799 -> [w810 _]
                tunnel: w798 -> [_ w814]
                tunnel: ["There was a crash!!!!" ("GUI Item Name") "Runs stopped!" ("Text to log")] -> w782
                tunnel: ["Skipping everything, clearing the queue" ("initial string") "STOPPED! Skipping everything, clearing the queue" ("initial string")] -> w797
                tunnel: [w810 w814] -> w796
                tunnel: w795 -> [w807 w813]
                tunnel: [w807 w813] -> w794
                tunnel: w793 -> [w806 w812]
                tunnel: [w806 w812] -> w792
                tunnel: [Monkey_Status."Finished (with errors)" ("Monkey Status") Monkey_Status."Stopped" ("Monkey Status")] -> w787
                frame False {
                  # "CRASH"
                }
                frame True {
                  # "STOP"
                }
              }
              n245 = Format Into String(format string=" %s %d. %s", error in=w792, "finished with error code:" ("initial string"), w796, w797) -> (resulting string=w803:string, error out=w804:errorcluster)  [unwired: 1 in]
              n246 = call "Update Report Previous RUNs.vi"("error in (no error)"=w804, "Previous RUN outcome"=w803, "Monkey in"=w794) -> ("error out"=w788:errorcluster, "Monkey out"=w789:refnum<class "Monkey.lvclass">)  [unwired: 7 in]
              n247 = call-dynamic "Skip all.vi"("error in (no error)"=w788, "Monkey in"=w789) -> ("error out"=w785:errorcluster, "Monkey out"=w786:refnum<class "Monkey.lvclass">)  [unwired: 8 in]
              n248 = call-dynamic "All RUNs Completed.vi"("error in (no error)"=w785, "Monkey in"=w786) -> ("error out"=w783:errorcluster, "Monkey out"=w784:refnum<class "Monkey.lvclass">)  [unwired: 7 in, 1 out]
              n249 = call "Update GUI.vi"("error in (no error)"=w783, "Data"=w782, "GUI Item Name"="Current Action", "uService Template in"=w784) -> ("error out"=w790:errorcluster, "uService Template out"=w791:refnum<class "Monkey.lvclass">)  [unwired: 6 in]
            }
            frame 4 {
              # "Something went horribly wrong, ABORT everything and run for your life"
              n250 = Format Into String(format string=" %s %d. %s", error in=w823, "finished with error code:" ("initial string"), w830, "Skipping everything!! ABORT!!" ("initial string")) -> (resulting string=w834:string, error out=w835:errorcluster)  [unwired: 1 in]
              n251 = call "Update Report Previous RUNs.vi"("error in (no error)"=w835, "Previous RUN outcome"=w834, "Monkey in"=w824) -> ("error out"=w826:errorcluster, "Monkey out"=w827:refnum<class "Monkey.lvclass">)  [unwired: 7 in]
              n252 = call-dynamic "Skip all.vi"("error in (no error)"=w826, "Monkey in"=w827) -> ("error out"=w817:errorcluster, "Monkey out"=w820:refnum<class "Monkey.lvclass">)  [unwired: 8 in]
              n253 = call-dynamic "All RUNs Completed.vi"("error in (no error)"=w817, "Monkey in"=w820) -> ("error out"=w818:errorcluster, "Monkey out"=w819:refnum<class "Monkey.lvclass">)  [unwired: 7 in, 1 out]
              n254 = call "Update GUI.vi"("error in (no error)"=w818, "Data"="Something went horribly wrong!!!!" ("GUI Item Name"), "GUI Item Name"="Current Action", "uService Template in"=w819) -> ("error out"=w822:errorcluster, "uService Template out"=w825:refnum<class "Monkey.lvclass">)  [unwired: 6 in]
            }
          }
          n255 = call-dynamic "Report to the Control uService.vi"("Monkey Status"=w622, "Monkey in"=w623) -> ("error out"=w621:errorcluster, "Monkey out"=w629:refnum<class "Monkey.lvclass">)  [unwired: 8 in]
          n256 = Merge Errors(w621, w620) -> (w628:errorcluster)
        }
        frame "Update Crit Lvl" {
          # "Should it be 3 or 0?\nIf someone forgets to put error criticality in the file, then we can assume it is 0. It is safer to keep as 3 though"
          # "If there was an error in variant to data, it means that the variant was empty: no specific error was provided. Ignore that error"
          # "Stop or ABORT?\nThis is handled by Tamer now. Monkey only deals with 0,1,2"
          n257 = global read "Global Constants.vi" "ABORT Crt Lvl"() -> (w847:u8)
          n258 = Variant To Data(error in=w859, type=u8 0, Variant=w860) -> (data=w852:u8, error out=w853:errorcluster)
          n259 = case shown="No Error" w853 {
            selector: w853 -> [w870 w875]
            tunnel: w852 -> [w871 _]
            tunnel: [w871 w872] -> w851
            tunnel: [w870 w874] -> w850
            tunnel: w847 -> [_ w873]
            frame No Error {
            }
            frame Error {
              n260 = call <vilib>:"Clear Errors.vi"("error in (no error)"=w875) -> ("error out"=w874:errorcluster)  [unwired: 5 in, 1 out]
              n261 = Decrement(x=w873) -> (x-1=w872:u8)
            }
          }
          n262 = In Range and Coerce(upper limit=w847, x=w851, lower limit=u8 0) -> (In Range?=w843:bool)  [unwired: 1 out]
          n263 = case shown="False" w843 {
            tunnel: w851 -> [_ w866]
            tunnel: w850 -> [_ w865]
            tunnel: [w864 w865] -> w856
            tunnel: [w862 w866] -> w858
            tunnel: w847 -> [w862 _]
            tunnel: w845 -> [w861 _]
            frame False {
              # "#5702"
              n264 = call "Generate Error.vi"("Class"=w861, "Error Code"=5702) -> ("error out"=w864:errorcluster)  [unwired: 5 in]
            }
            frame True {
              # "All good!"
            }
          }
          n265 = in-place {
            in-place-border: w858 -> [w867]
            in-place-border: [w869] -> w849
            n266 = in-place-cluster #2(w845) -> ("Criticality Level"=w868:u8)
            n267 = Max & Min(x=w868, y=w867) -> (max(x,y)=w869:u8)  [unwired: 1 out]
            n268 = in-place-cluster #2("Criticality Level"=w869) -> (w857:refnum<class "Monkey.lvclass">)
          }
          n269 = call "Update GUI.vi"("error in (no error)"=w856, "Data"=w849, "GUI Item Name"="Error Criticality", "uService Template in"=w857) -> ("error out"=w854:errorcluster, "uService Template out"=w855:refnum<class "Monkey.lvclass">)  [unwired: 6 in]
        }
        frame "Skip Run" {
          w886 = FALSE
          n270 = property class="Monkey.lvclass"(reference=w880) -> (reference out=w879:refnum<class "Monkey.lvclass">, "Accessors:STOPPED"=w877:bool)  [unwired: 1 in, 1 out]
          n271 = Variant To Data(type=w886, Variant=w884) -> (data=w887:bool, error out=w888:errorcluster)  [unwired: 1 in]
          n272 = Select(t=w886, s=w888, f=w887) -> (s? t:f=w885:bool)
          n273 = call-dynamic "Get FPGA uService ID.vi"("Monkey in"=w879) -> ("FPGA uService ID"=w881:string, "Monkey out"=w889:refnum<class "Monkey.lvclass">)  [unwired: 8 in, 1 out]
          n274 = Empty String/Path?(string/path=w881) -> (empty?=w878:bool)
          n275 = Or(x=w878, y=w877) -> (x .or. y?=w876:bool)
          n276 = case shown="False" w876 {
            tunnel: w890 -> [w904 w918]
            tunnel: w889 -> [w903 w919]
            tunnel: w881 -> [w891 _]
            tunnel: w885 -> [w902 _]
            tunnel: [w898 w919] -> w883
            tunnel: [w897 w918] -> w882
            frame False {
              n277 = call "Message to uService.vi"("Father of all uServices in"=w903, "uService ID"=w891, "Message"="Terminate Script", "Data"=w902, "error in (no error)"=w904) -> ("Father of all uServices out"=w901:refnum<class "Monkey.lvclass">, "error out"=w900:errorcluster)  [unwired: 9 in]
              n278 = case shown="False" w902 {
                tunnel: w901 -> [w912 w917]
                tunnel: w900 -> [w910 w916]
                tunnel: [w908 w917] -> w899
                tunnel: [w907 w916] -> w896
                tunnel: ["" w913] -> w894
                frame False {
                  # "Not gracefully, means we need to finish this Run manually"
                  n279 = call "Send to Consumer.vi"("error in (no error)"=w910, "Data"=u16 2, "Case ID"=Monkey_Consumer_Case_Selector."What to do next" ("Monkey Consumer Case Selector"), "uService Template in"=w912) -> ("error out"=w907:errorcluster, "uService Template out"=w908:refnum<class "Monkey.lvclass">)  [unwired: 6 in]
                }
                frame True {
                  # "Gracefully, the script's closure function will be executed and the"
                  n280 = call <vilib>:"Space Constant.vi"() -> ("String"=w914:string)
                  n281 = Concatenate Strings(w914, "(with grace)" ("GUI Item Name")) -> (w913:string)
                }
              }
              n282 = Concatenate Strings("Skipping script" ("string"), w894) -> (w893:string)
              n283 = call "Update GUI.vi"("error in (no error)"=w896, "Data"=w893, "GUI Item Name"="Current Action", "uService Template in"=w899) -> ("error out"=w897:errorcluster, "uService Template out"=w898:refnum<class "Monkey.lvclass">)  [unwired: 6 in]
            }
            frame True {
              # "Nothing to skip or stpped already"
            }
          }
        }
        frame "Stop Schedule" {
          w924 = T16 {"Old value"=FALSE, "Gracefully?"=FALSE} ("Stop msg")
          n284 = Variant To Data(type=w924, Variant=w930) -> (data=w933:T16, error out=w934:errorcluster)  [unwired: 1 in]
          n285 = Select(t=w924, s=w934, f=w933) -> (s? t:f=w923:T16)
          n286 = Unbundle By Name(w923) -> ("Old value"=w922:bool, "Gracefully?"=w921:bool)
          n287 = call-dynamic "Get FPGA uService ID.vi"("Monkey in"=w920) -> ("FPGA uService ID"=w926:string, "Monkey out"=w931:refnum<class "Monkey.lvclass">)  [unwired: 8 in, 1 out]
          n288 = Empty String/Path?(string/path=w926) -> (empty?=w925:bool)
          n289 = Or(x=w925, y=w922) -> (x .or. y?=w927:bool)
          n290 = case shown="False" w927 {
            tunnel: w932 -> [w948 w962]
            tunnel: w931 -> [w946 w963]
            tunnel: w926 -> [w945 _]
            tunnel: w921 -> [w944 _]
            tunnel: [w940 w963] -> w929
            tunnel: [w939 w962] -> w928
            frame False {
              n291 = call "Message to uService.vi"("Father of all uServices in"=w946, "uService ID"=w945, "Message"="Terminate Script", "Data"=w944, "error in (no error)"=w948) -> ("Father of all uServices out"=w943:refnum<class "Monkey.lvclass">, "error out"=w942:errorcluster)  [unwired: 9 in]
              n292 = case shown="False" w944 {
                tunnel: w943 -> [w956 w961]
                tunnel: w942 -> [w954 w960]
                tunnel: [w952 w961] -> w941
                tunnel: [w951 w960] -> w938
                tunnel: ["" w957] -> w936
                frame False {
                  # "Not gracefully, means we need to finish this Run manually"
                  n293 = call "Send to Consumer.vi"("error in (no error)"=w954, "Data"=u16 3, "Case ID"=Monkey_Consumer_Case_Selector."What to do next" ("Monkey Consumer Case Selector"), "uService Template in"=w956) -> ("error out"=w951:errorcluster, "uService Template out"=w952:refnum<class "Monkey.lvclass">)  [unwired: 6 in]
                }
                frame True {
                  # "Gracefully, the script's closure function will be executed and the"
                  n294 = call <vilib>:"Space Constant.vi"() -> ("String"=w958:string)
                  n295 = Concatenate Strings(w958, "(with grace)" ("GUI Item Name")) -> (w957:string)
                }
              }
              n296 = Concatenate Strings("Stoppig Schedule" ("string"), w936) -> (w935:string)
              n297 = call "Update GUI.vi"("error in (no error)"=w938, "Data"=w935, "GUI Item Name"="Current Action", "uService Template in"=w941) -> ("error out"=w939:errorcluster, "uService Template out"=w940:refnum<class "Monkey.lvclass">)  [unwired: 6 in]
            }
            frame True {
              # "Nothing to stop"
            }
          }
        }
        frame "Skip schedule" {
          n298 = call-dynamic "Skip schedule.vi"("error in (no error)"=w973, "Monkey in"=w974) -> ("error out"=w971:errorcluster, "Monkey out"=w972:refnum<class "Monkey.lvclass">)  [unwired: 8 in]
          n299 = call "Update GUI.vi"("error in (no error)"=w971, "Data"=FALSE, "GUI Item Name"="Skip schedule", "uService Template in"=w972) -> ("error out"=w967:errorcluster, "uService Template out"=w966:refnum<class "Monkey.lvclass">)  [unwired: 6 in]
          n300 = call "Send to Consumer.vi"("error in (no error)"=w967, "Case ID"=Monkey_Consumer_Case_Selector."Update GUI" ("Monkey Consumer Case Selector"), "uService Template in"=w966) -> ("error out"=w965:errorcluster, "uService Template out"=w964:refnum<class "Monkey.lvclass">)  [unwired: 7 in]
        }
      }
    }
    frame Error {
    }
  }
  n301 = call-parent "Consumer.vi"("error in (no error)"=w6, "Data"="Data", "Case ID"="Case ID", "uService Template in"=w3) -> ("error out"=→"error out":errorcluster, "uService Template out"=→"Monkey out":refnum<class "Monkey.lvclass">)  [unwired: 6 in]
